vi "SLSC Update Channels State to Tree Control.vi"(0 "Property tree":refnum<vi>, 1 "Update Only?":bool, 5 "SLSC Output Tree":T1(array[cluster])=[{"Left Cell String"="SLSC-12001-030EE1BC-Mod8", "Child Text"=[], "Child Tag"="Device", "Item Indent"=0, "Child Only?"=FALSE, "Glyph Index"=28}, {"Left Cell String"="Commands", "Child Text"=[], "Child Tag"="Device/Commands", "Item Indent"=1, "Child Only?"=FALSE, "Glyph Index"=35}, {"Left Cell String"="NI.UpdateChannelConfiguration", "Child Text"=["", "", "", "", "", "", "Command..NI.UpdateChannelConfiguration", "Command to complete updating physical channel properties", "This command enables simultaneous updating of the functional state of the module's physical channel configuration. Simultaneous updating of the physical channels' properties prevents the register write commit order from creating unexpected channel configuration states. Run this command to make changes to physical channels' properties take effect."], "Child Tag"="Device/Commands/NI.UpdateChannelConfiguration", "Item Indent"=2, "Child Only?"=FALSE, "Glyph Index"=4}, {"Left Cell String"="NI.UpdateTestMode", "Child Text"=["", "", "", "", "", "", "Command..NI.UpdateTestMode", "Command to complete updating Test Mode properties", "This command enable simultaneous updating of the functional state of the module's Test Mode configuration. Run this command to make changes to Test Mode properties take effect."], "Child Tag"="Device/Commands/NI.UpdateTestMode", "Item Indent"=2, "Child Only?"=FALSE, "Glyph Index"=4}, {"Left Cell String"="NI.Acknowledge24VPowerFailed", "Child Text"=["", "", "", "", "", "", "Command..NI.Acknowledge24VPowerFailed", "Command to acknowledge a latched 24V power failure status", "This command tries to clear the module's latched true state for the NI.Status24V_PowerFailed property. This command will have no effect on the latched state if the NI.Status24V_PowerGood property is still false."], "Child Tag"="Device/Commands/NI.Acknowledge24VPowerFailed", "Item Indent"=2, "Child Only?"=FALSE, "Glyph Index"=4}, {"Left Cell String"="Properties", "Child Text"=[], "Child Tag"="Device/Properties", "Item Indent"=1, "Child Only?"=FALSE, "Glyph Index"=36}, {"Left Cell String"="NI.ModuleControllerVersion", "Child Text"=["17022812", "Read Only", "U32", "", "", "", "[3.860173E+8].R.U32..NI.ModuleControllerVersion", "Module Controller Version", "The version is the timestamp, in hexadecimal format, of the time the Module Controller was compiled."], "Child Tag"="Device/Properties/NI.ModuleControllerVersion", "Item Indent"=2, "Child Only?"=FALSE, "Glyph Index"=8}, {"Left Cell String"="NI.RearBufferState", "Child Text"=["0", "Read Only", "U32", "", "", "", "[0].R.U32..NI.RearBufferState", "Logic state of all rear I/O connector input buffers", "Reading this property retrieves the current logic state of the rear I/O connector input buffers. This retrieval is controlled through the software system so the actual sampling time of the inputs is not deterministic. The value at each bit position is a function of the logic state at the XJ2 pin and the corresponding line's direction and enable configuration. An enabled line configured as an input will drive the rear I/O connector input buffer to the same state as detected at the front I/O connector input buffer."], "Child Tag"="Device/Properties/NI.RearBufferState", "Item Indent"=2, "Child Only?"=FALSE, "Glyph Index"=8}, {"Left Cell String"="NI.FrontBufferState", "Child Text"=["0", "Read Only", "U32", "", "", "", "[0].R.U32..NI.FrontBufferState", "Logic state of all front I/O connector input buffers", "Reading this property retrieves the current logic state of the front I/O connector input buffers. This retrieval is controlled through the software system so the actual sampling time of the inputs is not deterministic. The value at each bit position is a function of the voltage at the module DSUB pin and the bank range and threshold configuration. An enabled line configured as an output may drive the front I/O connector input buffer to a specific voltage, depending on the bank supply voltage configuration, the line's output topology, and the line's logic state from the rear I/O connector input buffer."], "Child Tag"="Device/Properties/NI.FrontBufferState", "Item Indent"=2, "Child Only?"=FALSE, "Glyph Index"=8}, {"Left Cell String"="NI.Status24VPowerFailed", "Child Text"=["False", "Read Only", "Bool", "", "", "", "[0].R.Bool..NI.Status24VPowerFailed", "State of the latched failure status of the module's 24V rail from the SLSC Interface", "When the NI.Status24V_PowerGood becomes false, this property latches as true until it is reset by the NI.Status24V_FaultAcknowledge command is sent after NI.Status24V_PowerGood returns to true. If this property is true, then the supply voltage selection for both banks of the module has been forced off for a nonzero duration."], "Child Tag"="Device/Properties/NI.Status24VPowerFailed", "Item Indent"=2, "Child Only?"=FALSE, "Glyph Index"=8}, {"Left Cell String"="NI.Status24VPowerGood", "Child Text"=["True", "Read Only", "Bool", "", "", "", "[1].R.Bool..NI.Status24VPowerGood", "State of the 24V rail on the module from the SLSC Interface", "When the 24V rail from the SLSC Interface drops below the safe operating range for the module, this property is set to false. Simultaneously, to protect the module's output circuitry and to prevent the module front I/O connector outputs from glitching high, the supply voltage selection for both banks is forced off until the 24V rail recovers and is stable."], "Child Tag"="Device/Properties/NI.Status24VPowerGood", "Item Indent"=2, "Child Only?"=FALSE, "Glyph Index"=8}, {"Left Cell String"="NI.Status3_3VPowerGood", "Child Text"=["True", "Read Only", "Bool", "", "", "", "[1].R.Bool..NI.Status3_3VPowerGood", "State of the 3.3V rail from the SLSC Interface on the module", "This property will always be true on a correctly functioning module because the module CPLD requires the 3.3V rail from the SLSC Interface to operate."], "Child Tag"="Device/Properties/NI.Status3_3VPowerGood", "Item Indent"=2, "Child Only?"=FALSE, "Glyph Index"=8}, {"Left Cell String"="NI.TestModeEnable", "Child Text"=["False", "Read/Write", "Bool", "", "", "", "[0].RW.Bool..NI.TestModeEnable", "Enable for Test Mode", "Enable state for the module's Test Mode. When Test Mode is enabled, the module will output the values from the NI.TestModeValue property on the corresponding lines. Each line's respective direction and enable configuration will still apply when Test Mode is active. The data source of the lines is the only change when Test Mode is active. Changes to this property take effect after running the NI.TestModeUpdate command."], "Child Tag"="Device/Properties/NI.TestModeEnable", "Item Indent"=2, "Child Only?"=FALSE, "Glyph Index"=9}, {"Left Cell String"="NI.TestModeValue", "Child Text"=["0", "Read/Write", "U32", "", "", "", "[0].RW.U32..NI.TestModeValue", "Output logic states for use during Test Mode", "Output logic states for the module for use during Test Mode. The logic state corresponding to each line may be set independently of the other states. Changes to this property take effect after running the NI.TestModeUpdate command."], "Child Tag"="Device/Properties/NI.TestModeValue", "Item Indent"=2, "Child Only?"=FALSE, "Glyph Index"=9}, {"Left Cell String"="SLSC-12001-030EE1BC-Mod8/bank0", "Child Text"=[], "Child Tag"="Physical Channel/bank0", "Item Indent"=1, "Child Only?"=FALSE, "Glyph Index"=31}, {"Left Cell String"="Commands", "Child Text"=[], "Child Tag"="Physical Channel/bank0/Commands", "Item Indent"=2, "Child Only?"=FALSE, "Glyph Index"=35}, {"Left Cell String"="Properties", "Child Text"=[], "Child Tag"="Physical Channel/bank0/Properties", "Item Indent"=2, "Child Only?"=FALSE, "Glyph Index"=36}, {"Left Cell String"="NI.VsupSelect", "Child Text"=["[0]Vsup_Off", "Read/Write", "I32", "Enum", "NI.VsupSource", "[0]Vsup_Off;[1]Vsup_0;[2]Vsup_1;", "[0].RW.I32.bank0.NI.VsupSelect", "Voltage source selection", "Voltage source selection for this bank. Changes to this property take effect after running the NI.ChannelConfigurationUpdate command."], "Child Tag"="Physical Channel/bank0/Properties/NI.VsupSelect", "Item Indent"=3, "Child Only?"=FALSE, "Glyph Index"=9}, {"Left Cell String"="NI.RangeEnable5V", "Child Text"=["False", "Read/Write", "Bool", "", "", "", "[0].RW.Bool.bank0.NI.RangeEnable5V", "Voltage range selection", "Enable state for this bank's voltage range. When enabled, this bank uses the NI.InputThreshold5V for the input threshold. When disabled, this bank uses the NI.InputThreshold33V for the input threshold. Changes to this property take effect after running the NI.ChannelConfigurationUpdate command."], "Child Tag"="Physical Channel/bank0/Properties/NI.RangeEnable5V", "Item Indent"=3, "Child Only?"=FALSE, "Glyph Index"=9}, {"Left Cell String"="NI.InputThreshold5V", "Child Text"=["0.7", "Read/Write", "DBL", "", "", "", "[0.7].RW.DBL.bank0.NI.InputThreshold5V", "Input threshold voltage for the 5 V range", "Input threshold voltage for this bank when its NI.RangeEnable5V is true. Changes to this property take effect after running the NI.ChannelConfigurationUpdate command."], "Child Tag"="Physical Channel/bank0/Properties/NI.InputThreshold5V", "Item Indent"=3, "Child Only?"=FALSE, "Glyph Index"=9}, {"Left Cell String"="NI.InputThreshold33V", "Child Text"=["3.706", "Read/Write", "DBL", "", "", "", "[3.706].RW.DBL.bank0.NI.InputThreshold33V", "Input threshold voltage for the 33 V range", "Input threshold voltage for this bank when its NI.RangeEnable5V is false. Changes to this property take effect after running the NI.ChannelConfigurationUpdate command."], "Child Tag"="Physical Channel/bank0/Properties/NI.InputThreshold33V", "Item Indent"=3, "Child Only?"=FALSE, "Glyph Index"=9}, {"Left Cell String"="SLSC-12001-030EE1BC-Mod8/bank1", "Child Text"=[], "Child Tag"="Physical Channel/bank1", "Item Indent"=1, "Child Only?"=FALSE, "Glyph Index"=31}, {"Left Cell String"="Commands", "Child Text"=[], "Child Tag"="Physical Channel/bank1/Commands", "Item Indent"=2, "Child Only?"=FALSE, "Glyph Index"=35}, {"Left Cell String"="Properties", "Child Text"=[], "Child Tag"="Physical Channel/bank1/Properties", "Item Indent"=2, "Child Only?"=FALSE, "Glyph Index"=36}, {"Left Cell String"="NI.VsupSelect", "Child Text"=["[0]Vsup_Off", "Read/Write", "I32", "Enum", "NI.VsupSource", "[0]Vsup_Off;[1]Vsup_0;[2]Vsup_1;", "[0].RW.I32.bank1.NI.VsupSelect", "Voltage source selection", "Voltage source selection for this bank. Changes to this property take effect after running the NI.ChannelConfigurationUpdate command."], "Child Tag"="Physical Channel/bank1/Properties/NI.VsupSelect", "Item Indent"=3, "Child Only?"=FALSE, "Glyph Index"=9}, {"Left Cell String"="NI.RangeEnable5V", "Child Text"=["False", "Read/Write", "Bool", "", "", "", "[0].RW.Bool.bank1.NI.RangeEnable5V", "Voltage range selection", "Enable state for this bank's voltage range. When enabled, this bank uses the NI.InputThreshold5V for the input threshold. When disabled, this bank uses the NI.InputThreshold33V for the input threshold. Changes to this property take effect after running the NI.ChannelConfigurationUpdate command."], "Child Tag"="Physical Channel/bank1/Properties/NI.RangeEnable5V", "Item Indent"=3, "Child Only?"=FALSE, "Glyph Index"=9}, {"Left Cell String"="NI.InputThreshold5V", "Child Text"=["0.7", "Read/Write", "DBL", "", "", "", "[0.7].RW.DBL.bank1.NI.InputThreshold5V", "Input threshold voltage for the 5 V range", "Input threshold voltage for this bank when its NI.RangeEnable5V is true. Changes to this property take effect after running the NI.ChannelConfigurationUpdate command."], "Child Tag"="Physical Channel/bank1/Properties/NI.InputThreshold5V", "Item Indent"=3, "Child Only?"=FALSE, "Glyph Index"=9}, {"Left Cell String"="NI.InputThreshold33V", "Child Text"=["3.706", "Read/Write", "DBL", "", "", "", "[3.706].RW.DBL.bank1.NI.InputThreshold33V", "Input threshold voltage for the 33 V range", "Input threshold voltage for this bank when its NI.RangeEnable5V is false. Changes to this property take effect after running the NI.ChannelConfigurationUpdate command."], "Child Tag"="Physical Channel/bank1/Properties/NI.InputThreshold33V", "Item Indent"=3, "Child Only?"=FALSE, "Glyph Index"=9}, {"Left Cell String"="SLSC-12001-030EE1BC-Mod8/port0/line0", "Child Text"=[], "Child Tag"="Physical Channel/port0/line0", "Item Indent"=1, "Child Only?"=FALSE, "Glyph Index"=31}, {"Left Cell String"="Commands", "Child Text"=[], "Child Tag"="Physical Channel/port0/line0/Commands", "Item Indent"=2, "Child Only?"=FALSE, "Glyph Index"=35}, {"Left Cell String"="Properties", "Child Text"=[], "Child Tag"="Physical Channel/port0/line0/Properties", "Item Indent"=2, "Child Only?"=FALSE, "Glyph Index"=36}, {"Left Cell String"="NI.Line.Index", "Child Text"=["0", "Read Only", "U32", "", "", "", "[0].R.U32.port0/line0.NI.Line.Index", "Overall index of this DIO line in the module", "This is the index of this DIO line for the aggregate module properties: NI.FrontInputBufferState, NI.RearInputBufferState, and NI.TestModeValue."], "Child Tag"="Physical Channel/port0/line0/Properties/NI.Line.Index", "Item Indent"=3, "Child Only?"=FALSE, "Glyph Index"=8}, {"Left Cell String"="NI.Line.Direction", "Child Text"=["[0]Input", "Read/Write", "I32", "Enum", "NI.Line.Direction", "[0]Input;[1]Output_Source;[2]Output_Sink;[3]Output_PushPull;", "[0].RW.I32.port0/line0.NI.Line.Direction", "DIO line direction", "Line signal flow direction through the module, relative to the front I/O connector. This property is only used when the NI.ChannelEnable for this line is set to true. Changes to this property take effect after running the NI.ChannelConfigurationUpdate command."], "Child Tag"="Physical Channel/port0/line0/Properties/NI.Line.Direction", "Item Indent"=3, "Child Only?"=FALSE, "Glyph Index"=9}, {"Left Cell String"="NI.Line.Enable", "Child Text"=["False", "Read/Write", "Bool", "", "", "", "[0].RW.Bool.port0/line0.NI.Line.Enable", "DIO line output enable", "DIO output enable for one line. When a line is enabled, the input and output buffers for the front I/O connector and the rear I/O connector of the line are configured based on the NI.Line.Direction property. When a line is not enabled, the buffers for both the front I/O connector and the rear I/O connector are configured as inputs. Changes to this property take effect after running the NI.ChannelConfigurationUpdate command."], "Child Tag"="Physical Channel/port0/line0/Properties/NI.Line.Enable", "Item Indent"=3, "Child Only?"=FALSE, "Glyph Index"=9}, {"Left Cell String"="SLSC-12001-030EE1BC-Mod8/port0/line1", "Child Text"=[], "Child Tag"="Physical Channel/port0/line1", "Item Indent"=1, "Child Only?"=FALSE, "Glyph Index"=31}, {"Left Cell String"="Commands", "Child Text"=[], "Child Tag"="Physical Channel/port0/line1/Commands", "Item Indent"=2, "Child Only?"=FALSE, "Glyph Index"=35}, {"Left Cell String"="Properties", "Child Text"=[], "Child Tag"="Physical Channel/port0/line1/Properties", "Item Indent"=2, "Child Only?"=FALSE, "Glyph Index"=36}, {"Left Cell String"="NI.Line.Index", "Child Text"=["1", "Read Only", "U32", "", "", "", "[1].R.U32.port0/line1.NI.Line.Index", "Overall index of this DIO line in the module", "This is the index of this DIO line for the aggregate module properties: NI.FrontInputBufferState, NI.RearInputBufferState, and NI.TestModeValue."], "Child Tag"="Physical Channel/port0/line1/Properties/NI.Line.Index", "Item Indent"=3, "Child Only?"=FALSE, "Glyph Index"=8}, {"Left Cell String"="NI.Line.Direction", "Child Text"=["[0]Input", "Read/Write", "I32", "Enum", "NI.Line.Direction", "[0]Input;[1]Output_Source;[2]Output_Sink;[3]Output_PushPull;", "[0].RW.I32.port0/line1.NI.Line.Direction", "DIO line direction", "Line signal flow direction through the module, relative to the front I/O connector. This property is only used when the NI.ChannelEnable for this line is set to true. Changes to this property take effect after running the NI.ChannelConfigurationUpdate command."], "Child Tag"="Physical Channel/port0/line1/Properties/NI.Line.Direction", "Item Indent"=3, "Child Only?"=FALSE, "Glyph Index"=9}, {"Left Cell String"="NI.Line.Enable", "Child Text"=["False", "Read/Write", "Bool", "", "", "", "[0].RW.Bool.port0/line1.NI.Line.Enable", "DIO line output enable", "DIO output enable for one line. When a line is enabled, the input and output buffers for the front I/O connector and the rear I/O connector of the line are configured based on the NI.Line.Direction property. When a line is not enabled, the buffers for both the front I/O connector and the rear I/O connector are configured as inputs. Changes to this property take effect after running the NI.ChannelConfigurationUpdate command."], "Child Tag"="Physical Channel/port0/line1/Properties/NI.Line.Enable", "Item Indent"=3, "Child Only?"=FALSE, "Glyph Index"=9}, {"Left Cell String"="SLSC-12001-030EE1BC-Mod8/port0/line2", "Child Text"=[], "Child Tag"="Physical Channel/port0/line2", "Item Indent"=1, "Child Only?"=FALSE, "Glyph Index"=31}, {"Left Cell String"="Commands", "Child Text"=[], "Child Tag"="Physical Channel/port0/line2/Commands", "Item Indent"=2, "Child Only?"=FALSE, "Glyph Index"=35}, {"Left Cell String"="Properties", "Child Text"=[], "Child Tag"="Physical Channel/port0/line2/Properties", "Item Indent"=2, "Child Only?"=FALSE, "Glyph Index"=36}, {"Left Cell String"="NI.Line.Index", "Child Text"=["2", "Read Only", "U32", "", "", "", "[2].R.U32.port0/line2.NI.Line.Index", "Overall index of this DIO line in the module", "This is the index of this DIO line for the aggregate module properties: NI.FrontInputBufferState, NI.RearInputBufferState, and NI.TestModeValue."], "Child Tag"="Physical Channel/port0/line2/Properties/NI.Line.Index", "Item Indent"=3, "Child Only?"=FALSE, "Glyph Index"=8}, {"Left Cell String"="NI.Line.Direction", "Child Text"=["[0]Input", "Read/Write", "I32", "Enum", "NI.Line.Direction", "[0]Input;[1]Output_Source;[2]Output_Sink;[3]Output_PushPull;", "[0].RW.I32.port0/line2.NI.Line.Direction", "DIO line direction", "Line signal flow direction through the module, relative to the front I/O connector. This property is only used when the NI.ChannelEnable for this line is set to true. Changes to this property take effect after running the NI.ChannelConfigurationUpdate command."], "Child Tag"="Physical Channel/port0/line2/Properties/NI.Line.Direction", "Item Indent"=3, "Child Only?"=FALSE, "Glyph Index"=9}, {"Left Cell String"="NI.Line.Enable", "Child Text"=["False", "Read/Write", "Bool", "", "", "", "[0].RW.Bool.port0/line2.NI.Line.Enable", "DIO line output enable", "DIO output enable for one line. When a line is enabled, the input and output buffers for the front I/O connector and the rear I/O connector of the line are configured based on the NI.Line.Direction property. When a line is not enabled, the buffers for both the front I/O connector and the rear I/O connector are configured as inputs. Changes to this property take effect after running the NI.ChannelConfigurationUpdate command."], "Child Tag"="Physical Channel/port0/line2/Properties/NI.Line.Enable", "Item Indent"=3, "Child Only?"=FALSE, "Glyph Index"=9}, {"Left Cell String"="SLSC-12001-030EE1BC-Mod8/port0/line3", "Child Text"=[], "Child Tag"="Physical Channel/port0/line3", "Item Indent"=1, "Child Only?"=FALSE, "Glyph Index"=31}, {"Left Cell String"="Commands", "Child Text"=[], "Child Tag"="Physical Channel/port0/line3/Commands", "Item Indent"=2, "Child Only?"=FALSE, "Glyph Index"=35}, {"Left Cell String"="Properties", "Child Text"=[], "Child Tag"="Physical Channel/port0/line3/Properties", "Item Indent"=2, "Child Only?"=FALSE, "Glyph Index"=36}, {"Left Cell String"="NI.Line.Index", "Child Text"=["3", "Read Only", "U32", "", "", "", "[3].R.U32.port0/line3.NI.Line.Index", "Overall index of this DIO line in the module", "This is the index of this DIO line for the aggregate module properties: NI.FrontInputBufferState, NI.RearInputBufferState, and NI.TestModeValue."], "Child Tag"="Physical Channel/port0/line3/Properties/NI.Line.Index", "Item Indent"=3, "Child Only?"=FALSE, "Glyph Index"=8}, {"Left Cell String"="NI.Line.Direction", "Child Text"=["[0]Input", "Read/Write", "I32", "Enum", "NI.Line.Direction", "[0]Input;[1]Output_Source;[2]Output_Sink;[3]Output_PushPull;", "[0].RW.I32.port0/line3.NI.Line.Direction", "DIO line direction", "Line signal flow direction through the module, relative to the front I/O connector. This property is only used when the NI.ChannelEnable for this line is set to true. Changes to this property take effect after running the NI.ChannelConfigurationUpdate command."], "Child Tag"="Physical Channel/port0/line3/Properties/NI.Line.Direction", "Item Indent"=3, "Child Only?"=FALSE, "Glyph Index"=9}, {"Left Cell String"="NI.Line.Enable", "Child Text"=["False", "Read/Write", "Bool", "", "", "", "[0].RW.Bool.port0/line3.NI.Line.Enable", "DIO line output enable", "DIO output enable for one line. When a line is enabled, the input and output buffers for the front I/O connector and the rear I/O connector of the line are configured based on the NI.Line.Direction property. When a line is not enabled, the buffers for both the front I/O connector and the rear I/O connector are configured as inputs. Changes to this property take effect after running the NI.ChannelConfigurationUpdate command."], "Child Tag"="Physical Channel/port0/line3/Properties/NI.Line.Enable", "Item Indent"=3, "Child Only?"=FALSE, "Glyph Index"=9}, {"Left Cell String"="SLSC-12001-030EE1BC-Mod8/port0/line4", "Child Text"=[], "Child Tag"="Physical Channel/port0/line4", "Item Indent"=1, "Child Only?"=FALSE, "Glyph Index"=31}, {"Left Cell String"="Commands", "Child Text"=[], "Child Tag"="Physical Channel/port0/line4/Commands", "Item Indent"=2, "Child Only?"=FALSE, "Glyph Index"=35}, {"Left Cell String"="Properties", "Child Text"=[], "Child Tag"="Physical Channel/port0/line4/Properties", "Item Indent"=2, "Child Only?"=FALSE, "Glyph Index"=36}, {"Left Cell String"="NI.Line.Index", "Child Text"=["4", "Read Only", "U32", "", "", "", "[4].R.U32.port0/line4.NI.Line.Index", "Overall index of this DIO line in the module", "This is the index of this DIO line for the aggregate module properties: NI.FrontInputBufferState, NI.RearInputBufferState, and NI.TestModeValue."], "Child Tag"="Physical Channel/port0/line4/Properties/NI.Line.Index", "Item Indent"=3, "Child Only?"=FALSE, "Glyph Index"=8}, {"Left Cell String"="NI.Line.Direction", "Child Text"=["[0]Input", "Read/Write", "I32", "Enum", "NI.Line.Direction", "[0]Input;[1]Output_Source;[2]Output_Sink;[3]Output_PushPull;", "[0].RW.I32.port0/line4.NI.Line.Direction", "DIO line direction", "Line signal flow direction through the module, relative to the front I/O connector. This property is only used when the NI.ChannelEnable for this line is set to true. Changes to this property take effect after running the NI.ChannelConfigurationUpdate command."], "Child Tag"="Physical Channel/port0/line4/Properties/NI.Line.Direction", "Item Indent"=3, "Child Only?"=FALSE, "Glyph Index"=9}, {"Left Cell String"="NI.Line.Enable", "Child Text"=["False", "Read/Write", "Bool", "", "", "", "[0].RW.Bool.port0/line4.NI.Line.Enable", "DIO line output enable", "DIO output enable for one line. When a line is enabled, the input and output buffers for the front I/O connector and the rear I/O connector of the line are configured based on the NI.Line.Direction property. When a line is not enabled, the buffers for both the front I/O connector and the rear I/O connector are configured as inputs. Changes to this property take effect after running the NI.ChannelConfigurationUpdate command."], "Child Tag"="Physical Channel/port0/line4/Properties/NI.Line.Enable", "Item Indent"=3, "Child Only?"=FALSE, "Glyph Index"=9}, {"Left Cell String"="SLSC-12001-030EE1BC-Mod8/port0/line5", "Child Text"=[], "Child Tag"="Physical Channel/port0/line5", "Item Indent"=1, "Child Only?"=FALSE, "Glyph Index"=31}, {"Left Cell String"="Commands", "Child Text"=[], "Child Tag"="Physical Channel/port0/line5/Commands", "Item Indent"=2, "Child Only?"=FALSE, "Glyph Index"=35}, {"Left Cell String"="Properties", "Child Text"=[], "Child Tag"="Physical Channel/port0/line5/Properties", "Item Indent"=2, "Child Only?"=FALSE, "Glyph Index"=36}, {"Left Cell String"="NI.Line.Index", "Child Text"=["5", "Read Only", "U32", "", "", "", "[5].R.U32.port0/line5.NI.Line.Index", "Overall index of this DIO line in the module", "This is the index of this DIO line for the aggregate module properties: NI.FrontInputBufferState, NI.RearInputBufferState, and NI.TestModeValue."], "Child Tag"="Physical Channel/port0/line5/Properties/NI.Line.Index", "Item Indent"=3, "Child Only?"=FALSE, "Glyph Index"=8}, {"Left Cell String"="NI.Line.Direction", "Child Text"=["[0]Input", "Read/Write", "I32", "Enum", "NI.Line.Direction", "[0]Input;[1]Output_Source;[2]Output_Sink;[3]Output_PushPull;", "[0].RW.I32.port0/line5.NI.Line.Direction", "DIO line direction", "Line signal flow direction through the module, relative to the front I/O connector. This property is only used when the NI.ChannelEnable for this line is set to true. Changes to this property take effect after running the NI.ChannelConfigurationUpdate command."], "Child Tag"="Physical Channel/port0/line5/Properties/NI.Line.Direction", "Item Indent"=3, "Child Only?"=FALSE, "Glyph Index"=9}, {"Left Cell String"="NI.Line.Enable", "Child Text"=["False", "Read/Write", "Bool", "", "", "", "[0].RW.Bool.port0/line5.NI.Line.Enable", "DIO line output enable", "DIO output enable for one line. When a line is enabled, the input and output buffers for the front I/O connector and the rear I/O connector of the line are configured based on the NI.Line.Direction property. When a line is not enabled, the buffers for both the front I/O connector and the rear I/O connector are configured as inputs. Changes to this property take effect after running the NI.ChannelConfigurationUpdate command."], "Child Tag"="Physical Channel/port0/line5/Properties/NI.Line.Enable", "Item Indent"=3, "Child Only?"=FALSE, "Glyph Index"=9}, {"Left Cell String"="SLSC-12001-030EE1BC-Mod8/port0/line6", "Child Text"=[], "Child Tag"="Physical Channel/port0/line6", "Item Indent"=1, "Child Only?"=FALSE, "Glyph Index"=31}, {"Left Cell String"="Commands", "Child Text"=[], "Child Tag"="Physical Channel/port0/line6/Commands", "Item Indent"=2, "Child Only?"=FALSE, "Glyph Index"=35}, {"Left Cell String"="Properties", "Child Text"=[], "Child Tag"="Physical Channel/port0/line6/Properties", "Item Indent"=2, "Child Only?"=FALSE, "Glyph Index"=36}, {"Left Cell String"="NI.Line.Index", "Child Text"=["6", "Read Only", "U32", "", "", "", "[6].R.U32.port0/line6.NI.Line.Index", "Overall index of this DIO line in the module", "This is the index of this DIO line for the aggregate module properties: NI.FrontInputBufferState, NI.RearInputBufferState, and NI.TestModeValue."], "Child Tag"="Physical Channel/port0/line6/Properties/NI.Line.Index", "Item Indent"=3, "Child Only?"=FALSE, "Glyph Index"=8}, {"Left Cell String"="NI.Line.Direction", "Child Text"=["[0]Input", "Read/Write", "I32", "Enum", "NI.Line.Direction", "[0]Input;[1]Output_Source;[2]Output_Sink;[3]Output_PushPull;", "[0].RW.I32.port0/line6.NI.Line.Direction", "DIO line direction", "Line signal flow direction through the module, relative to the front I/O connector. This property is only used when the NI.ChannelEnable for this line is set to true. Changes to this property take effect after running the NI.ChannelConfigurationUpdate command."], "Child Tag"="Physical Channel/port0/line6/Properties/NI.Line.Direction", "Item Indent"=3, "Child Only?"=FALSE, "Glyph Index"=9}, {"Left Cell String"="NI.Line.Enable", "Child Text"=["False", "Read/Write", "Bool", "", "", "", "[0].RW.Bool.port0/line6.NI.Line.Enable", "DIO line output enable", "DIO output enable for one line. When a line is enabled, the input and output buffers for the front I/O connector and the rear I/O connector of the line are configured based on the NI.Line.Direction property. When a line is not enabled, the buffers for both the front I/O connector and the rear I/O connector are configured as inputs. Changes to this property take effect after running the NI.ChannelConfigurationUpdate command."], "Child Tag"="Physical Channel/port0/line6/Properties/NI.Line.Enable", "Item Indent"=3, "Child Only?"=FALSE, "Glyph Index"=9}, {"Left Cell String"="SLSC-12001-030EE1BC-Mod8/port0/line7", "Child Text"=[], "Child Tag"="Physical Channel/port0/line7", "Item Indent"=1, "Child Only?"=FALSE, "Glyph Index"=31}, {"Left Cell String"="Commands", "Child Text"=[], "Child Tag"="Physical Channel/port0/line7/Commands", "Item Indent"=2, "Child Only?"=FALSE, "Glyph Index"=35}, {"Left Cell String"="Properties", "Child Text"=[], "Child Tag"="Physical Channel/port0/line7/Properties", "Item Indent"=2, "Child Only?"=FALSE, "Glyph Index"=36}, {"Left Cell String"="NI.Line.Index", "Child Text"=["7", "Read Only", "U32", "", "", "", "[7].R.U32.port0/line7.NI.Line.Index", "Overall index of this DIO line in the module", "This is the index of this DIO line for the aggregate module properties: NI.FrontInputBufferState, NI.RearInputBufferState, and NI.TestModeValue."], "Child Tag"="Physical Channel/port0/line7/Properties/NI.Line.Index", "Item Indent"=3, "Child Only?"=FALSE, "Glyph Index"=8}, {"Left Cell String"="NI.Line.Direction", "Child Text"=["[0]Input", "Read/Write", "I32", "Enum", "NI.Line.Direction", "[0]Input;[1]Output_Source;[2]Output_Sink;[3]Output_PushPull;", "[0].RW.I32.port0/line7.NI.Line.Direction", "DIO line direction", "Line signal flow direction through the module, relative to the front I/O connector. This property is only used when the NI.ChannelEnable for this line is set to true. Changes to this property take effect after running the NI.ChannelConfigurationUpdate command."], "Child Tag"="Physical Channel/port0/line7/Properties/NI.Line.Direction", "Item Indent"=3, "Child Only?"=FALSE, "Glyph Index"=9}, {"Left Cell String"="NI.Line.Enable", "Child Text"=["False", "Read/Write", "Bool", "", "", "", "[0].RW.Bool.port0/line7.NI.Line.Enable", "DIO line output enable", "DIO output enable for one line. When a line is enabled, the input and output buffers for the front I/O connector and the rear I/O connector of the line are configured based on the NI.Line.Direction property. When a line is not enabled, the buffers for both the front I/O connector and the rear I/O connector are configured as inputs. Changes to this property take effect after running the NI.ChannelConfigurationUpdate command."], "Child Tag"="Physical Channel/port0/line7/Properties/NI.Line.Enable", "Item Indent"=3, "Child Only?"=FALSE, "Glyph Index"=9}, {"Left Cell String"="SLSC-12001-030EE1BC-Mod8/port1/line0", "Child Text"=[], "Child Tag"="Physical Channel/port1/line0", "Item Indent"=1, "Child Only?"=FALSE, "Glyph Index"=31}, {"Left Cell String"="Commands", "Child Text"=[], "Child Tag"="Physical Channel/port1/line0/Commands", "Item Indent"=2, "Child Only?"=FALSE, "Glyph Index"=35}, {"Left Cell String"="Properties", "Child Text"=[], "Child Tag"="Physical Channel/port1/line0/Properties", "Item Indent"=2, "Child Only?"=FALSE, "Glyph Index"=36}, {"Left Cell String"="NI.Line.Index", "Child Text"=["8", "Read Only", "U32", "", "", "", "[8].R.U32.port1/line0.NI.Line.Index", "Overall index of this DIO line in the module", "This is the index of this DIO line for the aggregate module properties: NI.FrontInputBufferState, NI.RearInputBufferState, and NI.TestModeValue."], "Child Tag"="Physical Channel/port1/line0/Properties/NI.Line.Index", "Item Indent"=3, "Child Only?"=FALSE, "Glyph Index"=8}, {"Left Cell String"="NI.Line.Direction", "Child Text"=["[0]Input", "Read/Write", "I32", "Enum", "NI.Line.Direction", "[0]Input;[1]Output_Source;[2]Output_Sink;[3]Output_PushPull;", "[0].RW.I32.port1/line0.NI.Line.Direction", "DIO line direction", "Line signal flow direction through the module, relative to the front I/O connector. This property is only used when the NI.ChannelEnable for this line is set to true. Changes to this property take effect after running the NI.ChannelConfigurationUpdate command."], "Child Tag"="Physical Channel/port1/line0/Properties/NI.Line.Direction", "Item Indent"=3, "Child Only?"=FALSE, "Glyph Index"=9}, {"Left Cell String"="NI.Line.Enable", "Child Text"=["False", "Read/Write", "Bool", "", "", "", "[0].RW.Bool.port1/line0.NI.Line.Enable", "DIO line output enable", "DIO output enable for one line. When a line is enabled, the input and output buffers for the front I/O connector and the rear I/O connector of the line are configured based on the NI.Line.Direction property. When a line is not enabled, the buffers for both the front I/O connector and the rear I/O connector are configured as inputs. Changes to this property take effect after running the NI.ChannelConfigurationUpdate command."], "Child Tag"="Physical Channel/port1/line0/Properties/NI.Line.Enable", "Item Indent"=3, "Child Only?"=FALSE, "Glyph Index"=9}, {"Left Cell String"="SLSC-12001-030EE1BC-Mod8/port1/line1", "Child Text"=[], "Child Tag"="Physical Channel/port1/line1", "Item Indent"=1, "Child Only?"=FALSE, "Glyph Index"=31}, {"Left Cell String"="Commands", "Child Text"=[], "Child Tag"="Physical Channel/port1/line1/Commands", "Item Indent"=2, "Child Only?"=FALSE, "Glyph Index"=35}, {"Left Cell String"="Properties", "Child Text"=[], "Child Tag"="Physical Channel/port1/line1/Properties", "Item Indent"=2, "Child Only?"=FALSE, "Glyph Index"=36}, {"Left Cell String"="NI.Line.Index", "Child Text"=["9", "Read Only", "U32", "", "", "", "[9].R.U32.port1/line1.NI.Line.Index", "Overall index of this DIO line in the module", "This is the index of this DIO line for the aggregate module properties: NI.FrontInputBufferState, NI.RearInputBufferState, and NI.TestModeValue."], "Child Tag"="Physical Channel/port1/line1/Properties/NI.Line.Index", "Item Indent"=3, "Child Only?"=FALSE, "Glyph Index"=8}, {"Left Cell String"="NI.Line.Direction", "Child Text"=["[0]Input", "Read/Write", "I32", "Enum", "NI.Line.Direction", "[0]Input;[1]Output_Source;[2]Output_Sink;[3]Output_PushPull;", "[0].RW.I32.port1/line1.NI.Line.Direction", "DIO line direction", "Line signal flow direction through the module, relative to the front I/O connector. This property is only used when the NI.ChannelEnable for this line is set to true. Changes to this property take effect after running the NI.ChannelConfigurationUpdate command."], "Child Tag"="Physical Channel/port1/line1/Properties/NI.Line.Direction", "Item Indent"=3, "Child Only?"=FALSE, "Glyph Index"=9}, {"Left Cell String"="NI.Line.Enable", "Child Text"=["False", "Read/Write", "Bool", "", "", "", "[0].RW.Bool.port1/line1.NI.Line.Enable", "DIO line output enable", "DIO output enable for one line. When a line is enabled, the input and output buffers for the front I/O connector and the rear I/O connector of the line are configured based on the NI.Line.Direction property. When a line is not enabled, the buffers for both the front I/O connector and the rear I/O connector are configured as inputs. Changes to this property take effect after running the NI.ChannelConfigurationUpdate command."], "Child Tag"="Physical Channel/port1/line1/Properties/NI.Line.Enable", "Item Indent"=3, "Child Only?"=FALSE, "Glyph Index"=9}, {"Left Cell String"="SLSC-12001-030EE1BC-Mod8/port1/line2", "Child Text"=[], "Child Tag"="Physical Channel/port1/line2", "Item Indent"=1, "Child Only?"=FALSE, "Glyph Index"=31}, {"Left Cell String"="Commands", "Child Text"=[], "Child Tag"="Physical Channel/port1/line2/Commands", "Item Indent"=2, "Child Only?"=FALSE, "Glyph Index"=35}, {"Left Cell String"="Properties", "Child Text"=[], "Child Tag"="Physical Channel/port1/line2/Properties", "Item Indent"=2, "Child Only?"=FALSE, "Glyph Index"=36}, {"Left Cell String"="NI.Line.Index", "Child Text"=["A", "Read Only", "U32", "", "", "", "[10].R.U32.port1/line2.NI.Line.Index", "Overall index of this DIO line in the module", "This is the index of this DIO line for the aggregate module properties: NI.FrontInputBufferState, NI.RearInputBufferState, and NI.TestModeValue."], "Child Tag"="Physical Channel/port1/line2/Properties/NI.Line.Index", "Item Indent"=3, "Child Only?"=FALSE, "Glyph Index"=8}, {"Left Cell String"="NI.Line.Direction", "Child Text"=["[0]Input", "Read/Write", "I32", "Enum", "NI.Line.Direction", "[0]Input;[1]Output_Source;[2]Output_Sink;[3]Output_PushPull;", "[0].RW.I32.port1/line2.NI.Line.Direction", "DIO line direction", "Line signal flow direction through the module, relative to the front I/O connector. This property is only used when the NI.ChannelEnable for this line is set to true. Changes to this property take effect after running the NI.ChannelConfigurationUpdate command."], "Child Tag"="Physical Channel/port1/line2/Properties/NI.Line.Direction", "Item Indent"=3, "Child Only?"=FALSE, "Glyph Index"=9}, {"Left Cell String"="NI.Line.Enable", "Child Text"=["False", "Read/Write", "Bool", "", "", "", "[0].RW.Bool.port1/line2.NI.Line.Enable", "DIO line output enable", "DIO output enable for one line. When a line is enabled, the input and output buffers for the front I/O connector and the rear I/O connector of the line are configured based on the NI.Line.Direction property. When a line is not enabled, the buffers for both the front I/O connector and the rear I/O connector are configured as inputs. Changes to this property take effect after running the NI.ChannelConfigurationUpdate command."], "Child Tag"="Physical Channel/port1/line2/Properties/NI.Line.Enable", "Item Indent"=3, "Child Only?"=FALSE, "Glyph Index"=9}, {"Left Cell String"="SLSC-12001-030EE1BC-Mod8/port1/line3", "Child Text"=[], "Child Tag"="Physical Channel/port1/line3", "Item Indent"=1, "Child Only?"=FALSE, "Glyph Index"=31}, {"Left Cell String"="Commands", "Child Text"=[], "Child Tag"="Physical Channel/port1/line3/Commands", "Item Indent"=2, "Child Only?"=FALSE, "Glyph Index"=35}, {"Left Cell String"="Properties", "Child Text"=[], "Child Tag"="Physical Channel/port1/line3/Properties", "Item Indent"=2, "Child Only?"=FALSE, "Glyph Index"=36}, {"Left Cell String"="NI.Line.Index", "Child Text"=["B", "Read Only", "U32", "", "", "", "[11].R.U32.port1/line3.NI.Line.Index", "Overall index of this DIO line in the module", "This is the index of this DIO line for the aggregate module properties: NI.FrontInputBufferState, NI.RearInputBufferState, and NI.TestModeValue."], "Child Tag"="Physical Channel/port1/line3/Properties/NI.Line.Index", "Item Indent"=3, "Child Only?"=FALSE, "Glyph Index"=8}, {"Left Cell String"="NI.Line.Direction", "Child Text"=["[0]Input", "Read/Write", "I32", "Enum", "NI.Line.Direction", "[0]Input;[1]Output_Source;[2]Output_Sink;[3]Output_PushPull;", "[0].RW.I32.port1/line3.NI.Line.Direction", "DIO line direction", "Line signal flow direction through the module, relative to the front I/O connector. This property is only used when the NI.ChannelEnable for this line is set to true. Changes to this property take effect after running the NI.ChannelConfigurationUpdate command."], "Child Tag"="Physical Channel/port1/line3/Properties/NI.Line.Direction", "Item Indent"=3, "Child Only?"=FALSE, "Glyph Index"=9}, {"Left Cell String"="NI.Line.Enable", "Child Text"=["False", "Read/Write", "Bool", "", "", "", "[0].RW.Bool.port1/line3.NI.Line.Enable", "DIO line output enable", "DIO output enable for one line. When a line is enabled, the input and output buffers for the front I/O connector and the rear I/O connector of the line are configured based on the NI.Line.Direction property. When a line is not enabled, the buffers for both the front I/O connector and the rear I/O connector are configured as inputs. Changes to this property take effect after running the NI.ChannelConfigurationUpdate command."], "Child Tag"="Physical Channel/port1/line3/Properties/NI.Line.Enable", "Item Indent"=3, "Child Only?"=FALSE, "Glyph Index"=9}, {"Left Cell String"="SLSC-12001-030EE1BC-Mod8/port1/line4", "Child Text"=[], "Child Tag"="Physical Channel/port1/line4", "Item Indent"=1, "Child Only?"=FALSE, "Glyph Index"=31}, {"Left Cell String"="Commands", "Child Text"=[], "Child Tag"="Physical Channel/port1/line4/Commands", "Item Indent"=2, "Child Only?"=FALSE, "Glyph Index"=35}, {"Left Cell String"="Properties", "Child Text"=[], "Child Tag"="Physical Channel/port1/line4/Properties", "Item Indent"=2, "Child Only?"=FALSE, "Glyph Index"=36}, {"Left Cell String"="NI.Line.Index", "Child Text"=["C", "Read Only", "U32", "", "", "", "[12].R.U32.port1/line4.NI.Line.Index", "Overall index of this DIO line in the module", "This is the index of this DIO line for the aggregate module properties: NI.FrontInputBufferState, NI.RearInputBufferState, and NI.TestModeValue."], "Child Tag"="Physical Channel/port1/line4/Properties/NI.Line.Index", "Item Indent"=3, "Child Only?"=FALSE, "Glyph Index"=8}, {"Left Cell String"="NI.Line.Direction", "Child Text"=["[0]Input", "Read/Write", "I32", "Enum", "NI.Line.Direction", "[0]Input;[1]Output_Source;[2]Output_Sink;[3]Output_PushPull;", "[0].RW.I32.port1/line4.NI.Line.Direction", "DIO line direction", "Line signal flow direction through the module, relative to the front I/O connector. This property is only used when the NI.ChannelEnable for this line is set to true. Changes to this property take effect after running the NI.ChannelConfigurationUpdate command."], "Child Tag"="Physical Channel/port1/line4/Properties/NI.Line.Direction", "Item Indent"=3, "Child Only?"=FALSE, "Glyph Index"=9}, {"Left Cell String"="NI.Line.Enable", "Child Text"=["False", "Read/Write", "Bool", "", "", "", "[0].RW.Bool.port1/line4.NI.Line.Enable", "DIO line output enable", "DIO output enable for one line. When a line is enabled, the input and output buffers for the front I/O connector and the rear I/O connector of the line are configured based on the NI.Line.Direction property. When a line is not enabled, the buffers for both the front I/O connector and the rear I/O connector are configured as inputs. Changes to this property take effect after running the NI.ChannelConfigurationUpdate command."], "Child Tag"="Physical Channel/port1/line4/Properties/NI.Line.Enable", "Item Indent"=3, "Child Only?"=FALSE, "Glyph Index"=9}, {"Left Cell String"="SLSC-12001-030EE1BC-Mod8/port1/line5", "Child Text"=[], "Child Tag"="Physical Channel/port1/line5", "Item Indent"=1, "Child Only?"=FALSE, "Glyph Index"=31}, {"Left Cell String"="Commands", "Child Text"=[], "Child Tag"="Physical Channel/port1/line5/Commands", "Item Indent"=2, "Child Only?"=FALSE, "Glyph Index"=35}, {"Left Cell String"="Properties", "Child Text"=[], "Child Tag"="Physical Channel/port1/line5/Properties", "Item Indent"=2, "Child Only?"=FALSE, "Glyph Index"=36}, {"Left Cell String"="NI.Line.Index", "Child Text"=["D", "Read Only", "U32", "", "", "", "[13].R.U32.port1/line5.NI.Line.Index", "Overall index of this DIO line in the module", "This is the index of this DIO line for the aggregate module properties: NI.FrontInputBufferState, NI.RearInputBufferState, and NI.TestModeValue."], "Child Tag"="Physical Channel/port1/line5/Properties/NI.Line.Index", "Item Indent"=3, "Child Only?"=FALSE, "Glyph Index"=8}, {"Left Cell String"="NI.Line.Direction", "Child Text"=["[0]Input", "Read/Write", "I32", "Enum", "NI.Line.Direction", "[0]Input;[1]Output_Source;[2]Output_Sink;[3]Output_PushPull;", "[0].RW.I32.port1/line5.NI.Line.Direction", "DIO line direction", "Line signal flow direction through the module, relative to the front I/O connector. This property is only used when the NI.ChannelEnable for this line is set to true. Changes to this property take effect after running the NI.ChannelConfigurationUpdate command."], "Child Tag"="Physical Channel/port1/line5/Properties/NI.Line.Direction", "Item Indent"=3, "Child Only?"=FALSE, "Glyph Index"=9}, {"Left Cell String"="NI.Line.Enable", "Child Text"=["False", "Read/Write", "Bool", "", "", "", "[0].RW.Bool.port1/line5.NI.Line.Enable", "DIO line output enable", "DIO output enable for one line. When a line is enabled, the input and output buffers for the front I/O connector and the rear I/O connector of the line are configured based on the NI.Line.Direction property. When a line is not enabled, the buffers for both the front I/O connector and the rear I/O connector are configured as inputs. Changes to this property take effect after running the NI.ChannelConfigurationUpdate command."], "Child Tag"="Physical Channel/port1/line5/Properties/NI.Line.Enable", "Item Indent"=3, "Child Only?"=FALSE, "Glyph Index"=9}, {"Left Cell String"="SLSC-12001-030EE1BC-Mod8/port1/line6", "Child Text"=[], "Child Tag"="Physical Channel/port1/line6", "Item Indent"=1, "Child Only?"=FALSE, "Glyph Index"=31}, {"Left Cell String"="Commands", "Child Text"=[], "Child Tag"="Physical Channel/port1/line6/Commands", "Item Indent"=2, "Child Only?"=FALSE, "Glyph Index"=35}, {"Left Cell String"="Properties", "Child Text"=[], "Child Tag"="Physical Channel/port1/line6/Properties", "Item Indent"=2, "Child Only?"=FALSE, "Glyph Index"=36}, {"Left Cell String"="NI.Line.Index", "Child Text"=["E", "Read Only", "U32", "", "", "", "[14].R.U32.port1/line6.NI.Line.Index", "Overall index of this DIO line in the module", "This is the index of this DIO line for the aggregate module properties: NI.FrontInputBufferState, NI.RearInputBufferState, and NI.TestModeValue."], "Child Tag"="Physical Channel/port1/line6/Properties/NI.Line.Index", "Item Indent"=3, "Child Only?"=FALSE, "Glyph Index"=8}, {"Left Cell String"="NI.Line.Direction", "Child Text"=["[0]Input", "Read/Write", "I32", "Enum", "NI.Line.Direction", "[0]Input;[1]Output_Source;[2]Output_Sink;[3]Output_PushPull;", "[0].RW.I32.port1/line6.NI.Line.Direction", "DIO line direction", "Line signal flow direction through the module, relative to the front I/O connector. This property is only used when the NI.ChannelEnable for this line is set to true. Changes to this property take effect after running the NI.ChannelConfigurationUpdate command."], "Child Tag"="Physical Channel/port1/line6/Properties/NI.Line.Direction", "Item Indent"=3, "Child Only?"=FALSE, "Glyph Index"=9}, {"Left Cell String"="NI.Line.Enable", "Child Text"=["False", "Read/Write", "Bool", "", "", "", "[0].RW.Bool.port1/line6.NI.Line.Enable", "DIO line output enable", "DIO output enable for one line. When a line is enabled, the input and output buffers for the front I/O connector and the rear I/O connector of the line are configured based on the NI.Line.Direction property. When a line is not enabled, the buffers for both the front I/O connector and the rear I/O connector are configured as inputs. Changes to this property take effect after running the NI.ChannelConfigurationUpdate command."], "Child Tag"="Physical Channel/port1/line6/Properties/NI.Line.Enable", "Item Indent"=3, "Child Only?"=FALSE, "Glyph Index"=9}, {"Left Cell String"="SLSC-12001-030EE1BC-Mod8/port1/line7", "Child Text"=[], "Child Tag"="Physical Channel/port1/line7", "Item Indent"=1, "Child Only?"=FALSE, "Glyph Index"=31}, {"Left Cell String"="Commands", "Child Text"=[], "Child Tag"="Physical Channel/port1/line7/Commands", "Item Indent"=2, "Child Only?"=FALSE, "Glyph Index"=35}, {"Left Cell String"="Properties", "Child Text"=[], "Child Tag"="Physical Channel/port1/line7/Properties", "Item Indent"=2, "Child Only?"=FALSE, "Glyph Index"=36}, {"Left Cell String"="NI.Line.Index", "Child Text"=["F", "Read Only", "U32", "", "", "", "[15].R.U32.port1/line7.NI.Line.Index", "Overall index of this DIO line in the module", "This is the index of this DIO line for the aggregate module properties: NI.FrontInputBufferState, NI.RearInputBufferState, and NI.TestModeValue."], "Child Tag"="Physical Channel/port1/line7/Properties/NI.Line.Index", "Item Indent"=3, "Child Only?"=FALSE, "Glyph Index"=8}, {"Left Cell String"="NI.Line.Direction", "Child Text"=["[0]Input", "Read/Write", "I32", "Enum", "NI.Line.Direction", "[0]Input;[1]Output_Source;[2]Output_Sink;[3]Output_PushPull;", "[0].RW.I32.port1/line7.NI.Line.Direction", "DIO line direction", "Line signal flow direction through the module, relative to the front I/O connector. This property is only used when the NI.ChannelEnable for this line is set to true. Changes to this property take effect after running the NI.ChannelConfigurationUpdate command."], "Child Tag"="Physical Channel/port1/line7/Properties/NI.Line.Direction", "Item Indent"=3, "Child Only?"=FALSE, "Glyph Index"=9}, {"Left Cell String"="NI.Line.Enable", "Child Text"=["False", "Read/Write", "Bool", "", "", "", "[0].RW.Bool.port1/line7.NI.Line.Enable", "DIO line output enable", "DIO output enable for one line. When a line is enabled, the input and output buffers for the front I/O connector and the rear I/O connector of the line are configured based on the NI.Line.Direction property. When a line is not enabled, the buffers for both the front I/O connector and the rear I/O connector are configured as inputs. Changes to this property take effect after running the NI.ChannelConfigurationUpdate command."], "Child Tag"="Physical Channel/port1/line7/Properties/NI.Line.Enable", "Item Indent"=3, "Child Only?"=FALSE, "Glyph Index"=9}, {"Left Cell String"="SLSC-12001-030EE1BC-Mod8/port2/line0", "Child Text"=[], "Child Tag"="Physical Channel/port2/line0", "Item Indent"=1, "Child Only?"=FALSE, "Glyph Index"=31}, {"Left Cell String"="Commands", "Child Text"=[], "Child Tag"="Physical Channel/port2/line0/Commands", "Item Indent"=2, "Child Only?"=FALSE, "Glyph Index"=35}, {"Left Cell String"="Properties", "Child Text"=[], "Child Tag"="Physical Channel/port2/line0/Properties", "Item Indent"=2, "Child Only?"=FALSE, "Glyph Index"=36}, {"Left Cell String"="NI.Line.Index", "Child Text"=["10", "Read Only", "U32", "", "", "", "[16].R.U32.port2/line0.NI.Line.Index", "Overall index of this DIO line in the module", "This is the index of this DIO line for the aggregate module properties: NI.FrontInputBufferState, NI.RearInputBufferState, and NI.TestModeValue."], "Child Tag"="Physical Channel/port2/line0/Properties/NI.Line.Index", "Item Indent"=3, "Child Only?"=FALSE, "Glyph Index"=8}, {"Left Cell String"="NI.Line.Direction", "Child Text"=["[0]Input", "Read/Write", "I32", "Enum", "NI.Line.Direction", "[0]Input;[1]Output_Source;[2]Output_Sink;[3]Output_PushPull;", "[0].RW.I32.port2/line0.NI.Line.Direction", "DIO line direction", "Line signal flow direction through the module, relative to the front I/O connector. This property is only used when the NI.ChannelEnable for this line is set to true. Changes to this property take effect after running the NI.ChannelConfigurationUpdate command."], "Child Tag"="Physical Channel/port2/line0/Properties/NI.Line.Direction", "Item Indent"=3, "Child Only?"=FALSE, "Glyph Index"=9}, {"Left Cell String"="NI.Line.Enable", "Child Text"=["False", "Read/Write", "Bool", "", "", "", "[0].RW.Bool.port2/line0.NI.Line.Enable", "DIO line output enable", "DIO output enable for one line. When a line is enabled, the input and output buffers for the front I/O connector and the rear I/O connector of the line are configured based on the NI.Line.Direction property. When a line is not enabled, the buffers for both the front I/O connector and the rear I/O connector are configured as inputs. Changes to this property take effect after running the NI.ChannelConfigurationUpdate command."], "Child Tag"="Physical Channel/port2/line0/Properties/NI.Line.Enable", "Item Indent"=3, "Child Only?"=FALSE, "Glyph Index"=9}, {"Left Cell String"="SLSC-12001-030EE1BC-Mod8/port2/line1", "Child Text"=[], "Child Tag"="Physical Channel/port2/line1", "Item Indent"=1, "Child Only?"=FALSE, "Glyph Index"=31}, {"Left Cell String"="Commands", "Child Text"=[], "Child Tag"="Physical Channel/port2/line1/Commands", "Item Indent"=2, "Child Only?"=FALSE, "Glyph Index"=35}, {"Left Cell String"="Properties", "Child Text"=[], "Child Tag"="Physical Channel/port2/line1/Properties", "Item Indent"=2, "Child Only?"=FALSE, "Glyph Index"=36}, {"Left Cell String"="NI.Line.Index", "Child Text"=["11", "Read Only", "U32", "", "", "", "[17].R.U32.port2/line1.NI.Line.Index", "Overall index of this DIO line in the module", "This is the index of this DIO line for the aggregate module properties: NI.FrontInputBufferState, NI.RearInputBufferState, and NI.TestModeValue."], "Child Tag"="Physical Channel/port2/line1/Properties/NI.Line.Index", "Item Indent"=3, "Child Only?"=FALSE, "Glyph Index"=8}, {"Left Cell String"="NI.Line.Direction", "Child Text"=["[0]Input", "Read/Write", "I32", "Enum", "NI.Line.Direction", "[0]Input;[1]Output_Source;[2]Output_Sink;[3]Output_PushPull;", "[0].RW.I32.port2/line1.NI.Line.Direction", "DIO line direction", "Line signal flow direction through the module, relative to the front I/O connector. This property is only used when the NI.ChannelEnable for this line is set to true. Changes to this property take effect after running the NI.ChannelConfigurationUpdate command."], "Child Tag"="Physical Channel/port2/line1/Properties/NI.Line.Direction", "Item Indent"=3, "Child Only?"=FALSE, "Glyph Index"=9}, {"Left Cell String"="NI.Line.Enable", "Child Text"=["False", "Read/Write", "Bool", "", "", "", "[0].RW.Bool.port2/line1.NI.Line.Enable", "DIO line output enable", "DIO output enable for one line. When a line is enabled, the input and output buffers for the front I/O connector and the rear I/O connector of the line are configured based on the NI.Line.Direction property. When a line is not enabled, the buffers for both the front I/O connector and the rear I/O connector are configured as inputs. Changes to this property take effect after running the NI.ChannelConfigurationUpdate command."], "Child Tag"="Physical Channel/port2/line1/Properties/NI.Line.Enable", "Item Indent"=3, "Child Only?"=FALSE, "Glyph Index"=9}, {"Left Cell String"="SLSC-12001-030EE1BC-Mod8/port2/line2", "Child Text"=[], "Child Tag"="Physical Channel/port2/line2", "Item Indent"=1, "Child Only?"=FALSE, "Glyph Index"=31}, {"Left Cell String"="Commands", "Child Text"=[], "Child Tag"="Physical Channel/port2/line2/Commands", "Item Indent"=2, "Child Only?"=FALSE, "Glyph Index"=35}, {"Left Cell String"="Properties", "Child Text"=[], "Child Tag"="Physical Channel/port2/line2/Properties", "Item Indent"=2, "Child Only?"=FALSE, "Glyph Index"=36}, {"Left Cell String"="NI.Line.Index", "Child Text"=["12", "Read Only", "U32", "", "", "", "[18].R.U32.port2/line2.NI.Line.Index", "Overall index of this DIO line in the module", "This is the index of this DIO line for the aggregate module properties: NI.FrontInputBufferState, NI.RearInputBufferState, and NI.TestModeValue."], "Child Tag"="Physical Channel/port2/line2/Properties/NI.Line.Index", "Item Indent"=3, "Child Only?"=FALSE, "Glyph Index"=8}, {"Left Cell String"="NI.Line.Direction", "Child Text"=["[0]Input", "Read/Write", "I32", "Enum", "NI.Line.Direction", "[0]Input;[1]Output_Source;[2]Output_Sink;[3]Output_PushPull;", "[0].RW.I32.port2/line2.NI.Line.Direction", "DIO line direction", "Line signal flow direction through the module, relative to the front I/O connector. This property is only used when the NI.ChannelEnable for this line is set to true. Changes to this property take effect after running the NI.ChannelConfigurationUpdate command."], "Child Tag"="Physical Channel/port2/line2/Properties/NI.Line.Direction", "Item Indent"=3, "Child Only?"=FALSE, "Glyph Index"=9}, {"Left Cell String"="NI.Line.Enable", "Child Text"=["False", "Read/Write", "Bool", "", "", "", "[0].RW.Bool.port2/line2.NI.Line.Enable", "DIO line output enable", "DIO output enable for one line. When a line is enabled, the input and output buffers for the front I/O connector and the rear I/O connector of the line are configured based on the NI.Line.Direction property. When a line is not enabled, the buffers for both the front I/O connector and the rear I/O connector are configured as inputs. Changes to this property take effect after running the NI.ChannelConfigurationUpdate command."], "Child Tag"="Physical Channel/port2/line2/Properties/NI.Line.Enable", "Item Indent"=3, "Child Only?"=FALSE, "Glyph Index"=9}, {"Left Cell String"="SLSC-12001-030EE1BC-Mod8/port2/line3", "Child Text"=[], "Child Tag"="Physical Channel/port2/line3", "Item Indent"=1, "Child Only?"=FALSE, "Glyph Index"=31}, {"Left Cell String"="Commands", "Child Text"=[], "Child Tag"="Physical Channel/port2/line3/Commands", "Item Indent"=2, "Child Only?"=FALSE, "Glyph Index"=35}, {"Left Cell String"="Properties", "Child Text"=[], "Child Tag"="Physical Channel/port2/line3/Properties", "Item Indent"=2, "Child Only?"=FALSE, "Glyph Index"=36}, {"Left Cell String"="NI.Line.Index", "Child Text"=["13", "Read Only", "U32", "", "", "", "[19].R.U32.port2/line3.NI.Line.Index", "Overall index of this DIO line in the module", "This is the index of this DIO line for the aggregate module properties: NI.FrontInputBufferState, NI.RearInputBufferState, and NI.TestModeValue."], "Child Tag"="Physical Channel/port2/line3/Properties/NI.Line.Index", "Item Indent"=3, "Child Only?"=FALSE, "Glyph Index"=8}, {"Left Cell String"="NI.Line.Direction", "Child Text"=["[0]Input", "Read/Write", "I32", "Enum", "NI.Line.Direction", "[0]Input;[1]Output_Source;[2]Output_Sink;[3]Output_PushPull;", "[0].RW.I32.port2/line3.NI.Line.Direction", "DIO line direction", "Line signal flow direction through the module, relative to the front I/O connector. This property is only used when the NI.ChannelEnable for this line is set to true. Changes to this property take effect after running the NI.ChannelConfigurationUpdate command."], "Child Tag"="Physical Channel/port2/line3/Properties/NI.Line.Direction", "Item Indent"=3, "Child Only?"=FALSE, "Glyph Index"=9}, {"Left Cell String"="NI.Line.Enable", "Child Text"=["False", "Read/Write", "Bool", "", "", "", "[0].RW.Bool.port2/line3.NI.Line.Enable", "DIO line output enable", "DIO output enable for one line. When a line is enabled, the input and output buffers for the front I/O connector and the rear I/O connector of the line are configured based on the NI.Line.Direction property. When a line is not enabled, the buffers for both the front I/O connector and the rear I/O connector are configured as inputs. Changes to this property take effect after running the NI.ChannelConfigurationUpdate command."], "Child Tag"="Physical Channel/port2/line3/Properties/NI.Line.Enable", "Item Indent"=3, "Child Only?"=FALSE, "Glyph Index"=9}, {"Left Cell String"="SLSC-12001-030EE1BC-Mod8/port2/line4", "Child Text"=[], "Child Tag"="Physical Channel/port2/line4", "Item Indent"=1, "Child Only?"=FALSE, "Glyph Index"=31}, {"Left Cell String"="Commands", "Child Text"=[], "Child Tag"="Physical Channel/port2/line4/Commands", "Item Indent"=2, "Child Only?"=FALSE, "Glyph Index"=35}, {"Left Cell String"="Properties", "Child Text"=[], "Child Tag"="Physical Channel/port2/line4/Properties", "Item Indent"=2, "Child Only?"=FALSE, "Glyph Index"=36}, {"Left Cell String"="NI.Line.Index", "Child Text"=["14", "Read Only", "U32", "", "", "", "[20].R.U32.port2/line4.NI.Line.Index", "Overall index of this DIO line in the module", "This is the index of this DIO line for the aggregate module properties: NI.FrontInputBufferState, NI.RearInputBufferState, and NI.TestModeValue."], "Child Tag"="Physical Channel/port2/line4/Properties/NI.Line.Index", "Item Indent"=3, "Child Only?"=FALSE, "Glyph Index"=8}, {"Left Cell String"="NI.Line.Direction", "Child Text"=["[0]Input", "Read/Write", "I32", "Enum", "NI.Line.Direction", "[0]Input;[1]Output_Source;[2]Output_Sink;[3]Output_PushPull;", "[0].RW.I32.port2/line4.NI.Line.Direction", "DIO line direction", "Line signal flow direction through the module, relative to the front I/O connector. This property is only used when the NI.ChannelEnable for this line is set to true. Changes to this property take effect after running the NI.ChannelConfigurationUpdate command."], "Child Tag"="Physical Channel/port2/line4/Properties/NI.Line.Direction", "Item Indent"=3, "Child Only?"=FALSE, "Glyph Index"=9}, {"Left Cell String"="NI.Line.Enable", "Child Text"=["False", "Read/Write", "Bool", "", "", "", "[0].RW.Bool.port2/line4.NI.Line.Enable", "DIO line output enable", "DIO output enable for one line. When a line is enabled, the input and output buffers for the front I/O connector and the rear I/O connector of the line are configured based on the NI.Line.Direction property. When a line is not enabled, the buffers for both the front I/O connector and the rear I/O connector are configured as inputs. Changes to this property take effect after running the NI.ChannelConfigurationUpdate command."], "Child Tag"="Physical Channel/port2/line4/Properties/NI.Line.Enable", "Item Indent"=3, "Child Only?"=FALSE, "Glyph Index"=9}, {"Left Cell String"="SLSC-12001-030EE1BC-Mod8/port2/line5", "Child Text"=[], "Child Tag"="Physical Channel/port2/line5", "Item Indent"=1, "Child Only?"=FALSE, "Glyph Index"=31}, {"Left Cell String"="Commands", "Child Text"=[], "Child Tag"="Physical Channel/port2/line5/Commands", "Item Indent"=2, "Child Only?"=FALSE, "Glyph Index"=35}, {"Left Cell String"="Properties", "Child Text"=[], "Child Tag"="Physical Channel/port2/line5/Properties", "Item Indent"=2, "Child Only?"=FALSE, "Glyph Index"=36}, {"Left Cell String"="NI.Line.Index", "Child Text"=["15", "Read Only", "U32", "", "", "", "[21].R.U32.port2/line5.NI.Line.Index", "Overall index of this DIO line in the module", "This is the index of this DIO line for the aggregate module properties: NI.FrontInputBufferState, NI.RearInputBufferState, and NI.TestModeValue."], "Child Tag"="Physical Channel/port2/line5/Properties/NI.Line.Index", "Item Indent"=3, "Child Only?"=FALSE, "Glyph Index"=8}, {"Left Cell String"="NI.Line.Direction", "Child Text"=["[0]Input", "Read/Write", "I32", "Enum", "NI.Line.Direction", "[0]Input;[1]Output_Source;[2]Output_Sink;[3]Output_PushPull;", "[0].RW.I32.port2/line5.NI.Line.Direction", "DIO line direction", "Line signal flow direction through the module, relative to the front I/O connector. This property is only used when the NI.ChannelEnable for this line is set to true. Changes to this property take effect after running the NI.ChannelConfigurationUpdate command."], "Child Tag"="Physical Channel/port2/line5/Properties/NI.Line.Direction", "Item Indent"=3, "Child Only?"=FALSE, "Glyph Index"=9}, {"Left Cell String"="NI.Line.Enable", "Child Text"=["False", "Read/Write", "Bool", "", "", "", "[0].RW.Bool.port2/line5.NI.Line.Enable", "DIO line output enable", "DIO output enable for one line. When a line is enabled, the input and output buffers for the front I/O connector and the rear I/O connector of the line are configured based on the NI.Line.Direction property. When a line is not enabled, the buffers for both the front I/O connector and the rear I/O connector are configured as inputs. Changes to this property take effect after running the NI.ChannelConfigurationUpdate command."], "Child Tag"="Physical Channel/port2/line5/Properties/NI.Line.Enable", "Item Indent"=3, "Child Only?"=FALSE, "Glyph Index"=9}, {"Left Cell String"="SLSC-12001-030EE1BC-Mod8/port2/line6", "Child Text"=[], "Child Tag"="Physical Channel/port2/line6", "Item Indent"=1, "Child Only?"=FALSE, "Glyph Index"=31}, {"Left Cell String"="Commands", "Child Text"=[], "Child Tag"="Physical Channel/port2/line6/Commands", "Item Indent"=2, "Child Only?"=FALSE, "Glyph Index"=35}, {"Left Cell String"="Properties", "Child Text"=[], "Child Tag"="Physical Channel/port2/line6/Properties", "Item Indent"=2, "Child Only?"=FALSE, "Glyph Index"=36}, {"Left Cell String"="NI.Line.Index", "Child Text"=["16", "Read Only", "U32", "", "", "", "[22].R.U32.port2/line6.NI.Line.Index", "Overall index of this DIO line in the module", "This is the index of this DIO line for the aggregate module properties: NI.FrontInputBufferState, NI.RearInputBufferState, and NI.TestModeValue."], "Child Tag"="Physical Channel/port2/line6/Properties/NI.Line.Index", "Item Indent"=3, "Child Only?"=FALSE, "Glyph Index"=8}, {"Left Cell String"="NI.Line.Direction", "Child Text"=["[0]Input", "Read/Write", "I32", "Enum", "NI.Line.Direction", "[0]Input;[1]Output_Source;[2]Output_Sink;[3]Output_PushPull;", "[0].RW.I32.port2/line6.NI.Line.Direction", "DIO line direction", "Line signal flow direction through the module, relative to the front I/O connector. This property is only used when the NI.ChannelEnable for this line is set to true. Changes to this property take effect after running the NI.ChannelConfigurationUpdate command."], "Child Tag"="Physical Channel/port2/line6/Properties/NI.Line.Direction", "Item Indent"=3, "Child Only?"=FALSE, "Glyph Index"=9}, {"Left Cell String"="NI.Line.Enable", "Child Text"=["False", "Read/Write", "Bool", "", "", "", "[0].RW.Bool.port2/line6.NI.Line.Enable", "DIO line output enable", "DIO output enable for one line. When a line is enabled, the input and output buffers for the front I/O connector and the rear I/O connector of the line are configured based on the NI.Line.Direction property. When a line is not enabled, the buffers for both the front I/O connector and the rear I/O connector are configured as inputs. Changes to this property take effect after running the NI.ChannelConfigurationUpdate command."], "Child Tag"="Physical Channel/port2/line6/Properties/NI.Line.Enable", "Item Indent"=3, "Child Only?"=FALSE, "Glyph Index"=9}, {"Left Cell String"="SLSC-12001-030EE1BC-Mod8/port2/line7", "Child Text"=[], "Child Tag"="Physical Channel/port2/line7", "Item Indent"=1, "Child Only?"=FALSE, "Glyph Index"=31}, {"Left Cell String"="Commands", "Child Text"=[], "Child Tag"="Physical Channel/port2/line7/Commands", "Item Indent"=2, "Child Only?"=FALSE, "Glyph Index"=35}, {"Left Cell String"="Properties", "Child Text"=[], "Child Tag"="Physical Channel/port2/line7/Properties", "Item Indent"=2, "Child Only?"=FALSE, "Glyph Index"=36}, {"Left Cell String"="NI.Line.Index", "Child Text"=["17", "Read Only", "U32", "", "", "", "[23].R.U32.port2/line7.NI.Line.Index", "Overall index of this DIO line in the module", "This is the index of this DIO line for the aggregate module properties: NI.FrontInputBufferState, NI.RearInputBufferState, and NI.TestModeValue."], "Child Tag"="Physical Channel/port2/line7/Properties/NI.Line.Index", "Item Indent"=3, "Child Only?"=FALSE, "Glyph Index"=8}, {"Left Cell String"="NI.Line.Direction", "Child Text"=["[0]Input", "Read/Write", "I32", "Enum", "NI.Line.Direction", "[0]Input;[1]Output_Source;[2]Output_Sink;[3]Output_PushPull;", "[0].RW.I32.port2/line7.NI.Line.Direction", "DIO line direction", "Line signal flow direction through the module, relative to the front I/O connector. This property is only used when the NI.ChannelEnable for this line is set to true. Changes to this property take effect after running the NI.ChannelConfigurationUpdate command."], "Child Tag"="Physical Channel/port2/line7/Properties/NI.Line.Direction", "Item Indent"=3, "Child Only?"=FALSE, "Glyph Index"=9}, {"Left Cell String"="NI.Line.Enable", "Child Text"=["False", "Read/Write", "Bool", "", "", "", "[0].RW.Bool.port2/line7.NI.Line.Enable", "DIO line output enable", "DIO output enable for one line. When a line is enabled, the input and output buffers for the front I/O connector and the rear I/O connector of the line are configured based on the NI.Line.Direction property. When a line is not enabled, the buffers for both the front I/O connector and the rear I/O connector are configured as inputs. Changes to this property take effect after running the NI.ChannelConfigurationUpdate command."], "Child Tag"="Physical Channel/port2/line7/Properties/NI.Line.Enable", "Item Indent"=3, "Child Only?"=FALSE, "Glyph Index"=9}, {"Left Cell String"="SLSC-12001-030EE1BC-Mod8/port3/line0", "Child Text"=[], "Child Tag"="Physical Channel/port3/line0", "Item Indent"=1, "Child Only?"=FALSE, "Glyph Index"=31}, {"Left Cell String"="Commands", "Child Text"=[], "Child Tag"="Physical Channel/port3/line0/Commands", "Item Indent"=2, "Child Only?"=FALSE, "Glyph Index"=35}, {"Left Cell String"="Properties", "Child Text"=[], "Child Tag"="Physical Channel/port3/line0/Properties", "Item Indent"=2, "Child Only?"=FALSE, "Glyph Index"=36}, {"Left Cell String"="NI.Line.Index", "Child Text"=["18", "Read Only", "U32", "", "", "", "[24].R.U32.port3/line0.NI.Line.Index", "Overall index of this DIO line in the module", "This is the index of this DIO line for the aggregate module properties: NI.FrontInputBufferState, NI.RearInputBufferState, and NI.TestModeValue."], "Child Tag"="Physical Channel/port3/line0/Properties/NI.Line.Index", "Item Indent"=3, "Child Only?"=FALSE, "Glyph Index"=8}, {"Left Cell String"="NI.Line.Direction", "Child Text"=["[0]Input", "Read/Write", "I32", "Enum", "NI.Line.Direction", "[0]Input;[1]Output_Source;[2]Output_Sink;[3]Output_PushPull;", "[0].RW.I32.port3/line0.NI.Line.Direction", "DIO line direction", "Line signal flow direction through the module, relative to the front I/O connector. This property is only used when the NI.ChannelEnable for this line is set to true. Changes to this property take effect after running the NI.ChannelConfigurationUpdate command."], "Child Tag"="Physical Channel/port3/line0/Properties/NI.Line.Direction", "Item Indent"=3, "Child Only?"=FALSE, "Glyph Index"=9}, {"Left Cell String"="NI.Line.Enable", "Child Text"=["False", "Read/Write", "Bool", "", "", "", "[0].RW.Bool.port3/line0.NI.Line.Enable", "DIO line output enable", "DIO output enable for one line. When a line is enabled, the input and output buffers for the front I/O connector and the rear I/O connector of the line are configured based on the NI.Line.Direction property. When a line is not enabled, the buffers for both the front I/O connector and the rear I/O connector are configured as inputs. Changes to this property take effect after running the NI.ChannelConfigurationUpdate command."], "Child Tag"="Physical Channel/port3/line0/Properties/NI.Line.Enable", "Item Indent"=3, "Child Only?"=FALSE, "Glyph Index"=9}, {"Left Cell String"="SLSC-12001-030EE1BC-Mod8/port3/line1", "Child Text"=[], "Child Tag"="Physical Channel/port3/line1", "Item Indent"=1, "Child Only?"=FALSE, "Glyph Index"=31}, {"Left Cell String"="Commands", "Child Text"=[], "Child Tag"="Physical Channel/port3/line1/Commands", "Item Indent"=2, "Child Only?"=FALSE, "Glyph Index"=35}, {"Left Cell String"="Properties", "Child Text"=[], "Child Tag"="Physical Channel/port3/line1/Properties", "Item Indent"=2, "Child Only?"=FALSE, "Glyph Index"=36}, {"Left Cell String"="NI.Line.Index", "Child Text"=["19", "Read Only", "U32", "", "", "", "[25].R.U32.port3/line1.NI.Line.Index", "Overall index of this DIO line in the module", "This is the index of this DIO line for the aggregate module properties: NI.FrontInputBufferState, NI.RearInputBufferState, and NI.TestModeValue."], "Child Tag"="Physical Channel/port3/line1/Properties/NI.Line.Index", "Item Indent"=3, "Child Only?"=FALSE, "Glyph Index"=8}, {"Left Cell String"="NI.Line.Direction", "Child Text"=["[0]Input", "Read/Write", "I32", "Enum", "NI.Line.Direction", "[0]Input;[1]Output_Source;[2]Output_Sink;[3]Output_PushPull;", "[0].RW.I32.port3/line1.NI.Line.Direction", "DIO line direction", "Line signal flow direction through the module, relative to the front I/O connector. This property is only used when the NI.ChannelEnable for this line is set to true. Changes to this property take effect after running the NI.ChannelConfigurationUpdate command."], "Child Tag"="Physical Channel/port3/line1/Properties/NI.Line.Direction", "Item Indent"=3, "Child Only?"=FALSE, "Glyph Index"=9}, {"Left Cell String"="NI.Line.Enable", "Child Text"=["False", "Read/Write", "Bool", "", "", "", "[0].RW.Bool.port3/line1.NI.Line.Enable", "DIO line output enable", "DIO output enable for one line. When a line is enabled, the input and output buffers for the front I/O connector and the rear I/O connector of the line are configured based on the NI.Line.Direction property. When a line is not enabled, the buffers for both the front I/O connector and the rear I/O connector are configured as inputs. Changes to this property take effect after running the NI.ChannelConfigurationUpdate command."], "Child Tag"="Physical Channel/port3/line1/Properties/NI.Line.Enable", "Item Indent"=3, "Child Only?"=FALSE, "Glyph Index"=9}, {"Left Cell String"="SLSC-12001-030EE1BC-Mod8/port3/line2", "Child Text"=[], "Child Tag"="Physical Channel/port3/line2", "Item Indent"=1, "Child Only?"=FALSE, "Glyph Index"=31}, {"Left Cell String"="Commands", "Child Text"=[], "Child Tag"="Physical Channel/port3/line2/Commands", "Item Indent"=2, "Child Only?"=FALSE, "Glyph Index"=35}, {"Left Cell String"="Properties", "Child Text"=[], "Child Tag"="Physical Channel/port3/line2/Properties", "Item Indent"=2, "Child Only?"=FALSE, "Glyph Index"=36}, {"Left Cell String"="NI.Line.Index", "Child Text"=["1A", "Read Only", "U32", "", "", "", "[26].R.U32.port3/line2.NI.Line.Index", "Overall index of this DIO line in the module", "This is the index of this DIO line for the aggregate module properties: NI.FrontInputBufferState, NI.RearInputBufferState, and NI.TestModeValue."], "Child Tag"="Physical Channel/port3/line2/Properties/NI.Line.Index", "Item Indent"=3, "Child Only?"=FALSE, "Glyph Index"=8}, {"Left Cell String"="NI.Line.Direction", "Child Text"=["[0]Input", "Read/Write", "I32", "Enum", "NI.Line.Direction", "[0]Input;[1]Output_Source;[2]Output_Sink;[3]Output_PushPull;", "[0].RW.I32.port3/line2.NI.Line.Direction", "DIO line direction", "Line signal flow direction through the module, relative to the front I/O connector. This property is only used when the NI.ChannelEnable for this line is set to true. Changes to this property take effect after running the NI.ChannelConfigurationUpdate command."], "Child Tag"="Physical Channel/port3/line2/Properties/NI.Line.Direction", "Item Indent"=3, "Child Only?"=FALSE, "Glyph Index"=9}, {"Left Cell String"="NI.Line.Enable", "Child Text"=["False", "Read/Write", "Bool", "", "", "", "[0].RW.Bool.port3/line2.NI.Line.Enable", "DIO line output enable", "DIO output enable for one line. When a line is enabled, the input and output buffers for the front I/O connector and the rear I/O connector of the line are configured based on the NI.Line.Direction property. When a line is not enabled, the buffers for both the front I/O connector and the rear I/O connector are configured as inputs. Changes to this property take effect after running the NI.ChannelConfigurationUpdate command."], "Child Tag"="Physical Channel/port3/line2/Properties/NI.Line.Enable", "Item Indent"=3, "Child Only?"=FALSE, "Glyph Index"=9}, {"Left Cell String"="SLSC-12001-030EE1BC-Mod8/port3/line3", "Child Text"=[], "Child Tag"="Physical Channel/port3/line3", "Item Indent"=1, "Child Only?"=FALSE, "Glyph Index"=31}, {"Left Cell String"="Commands", "Child Text"=[], "Child Tag"="Physical Channel/port3/line3/Commands", "Item Indent"=2, "Child Only?"=FALSE, "Glyph Index"=35}, {"Left Cell String"="Properties", "Child Text"=[], "Child Tag"="Physical Channel/port3/line3/Properties", "Item Indent"=2, "Child Only?"=FALSE, "Glyph Index"=36}, {"Left Cell String"="NI.Line.Index", "Child Text"=["1B", "Read Only", "U32", "", "", "", "[27].R.U32.port3/line3.NI.Line.Index", "Overall index of this DIO line in the module", "This is the index of this DIO line for the aggregate module properties: NI.FrontInputBufferState, NI.RearInputBufferState, and NI.TestModeValue."], "Child Tag"="Physical Channel/port3/line3/Properties/NI.Line.Index", "Item Indent"=3, "Child Only?"=FALSE, "Glyph Index"=8}, {"Left Cell String"="NI.Line.Direction", "Child Text"=["[0]Input", "Read/Write", "I32", "Enum", "NI.Line.Direction", "[0]Input;[1]Output_Source;[2]Output_Sink;[3]Output_PushPull;", "[0].RW.I32.port3/line3.NI.Line.Direction", "DIO line direction", "Line signal flow direction through the module, relative to the front I/O connector. This property is only used when the NI.ChannelEnable for this line is set to true. Changes to this property take effect after running the NI.ChannelConfigurationUpdate command."], "Child Tag"="Physical Channel/port3/line3/Properties/NI.Line.Direction", "Item Indent"=3, "Child Only?"=FALSE, "Glyph Index"=9}, {"Left Cell String"="NI.Line.Enable", "Child Text"=["False", "Read/Write", "Bool", "", "", "", "[0].RW.Bool.port3/line3.NI.Line.Enable", "DIO line output enable", "DIO output enable for one line. When a line is enabled, the input and output buffers for the front I/O connector and the rear I/O connector of the line are configured based on the NI.Line.Direction property. When a line is not enabled, the buffers for both the front I/O connector and the rear I/O connector are configured as inputs. Changes to this property take effect after running the NI.ChannelConfigurationUpdate command."], "Child Tag"="Physical Channel/port3/line3/Properties/NI.Line.Enable", "Item Indent"=3, "Child Only?"=FALSE, "Glyph Index"=9}, {"Left Cell String"="SLSC-12001-030EE1BC-Mod8/port3/line4", "Child Text"=[], "Child Tag"="Physical Channel/port3/line4", "Item Indent"=1, "Child Only?"=FALSE, "Glyph Index"=31}, {"Left Cell String"="Commands", "Child Text"=[], "Child Tag"="Physical Channel/port3/line4/Commands", "Item Indent"=2, "Child Only?"=FALSE, "Glyph Index"=35}, {"Left Cell String"="Properties", "Child Text"=[], "Child Tag"="Physical Channel/port3/line4/Properties", "Item Indent"=2, "Child Only?"=FALSE, "Glyph Index"=36}, {"Left Cell String"="NI.Line.Index", "Child Text"=["1C", "Read Only", "U32", "", "", "", "[28].R.U32.port3/line4.NI.Line.Index", "Overall index of this DIO line in the module", "This is the index of this DIO line for the aggregate module properties: NI.FrontInputBufferState, NI.RearInputBufferState, and NI.TestModeValue."], "Child Tag"="Physical Channel/port3/line4/Properties/NI.Line.Index", "Item Indent"=3, "Child Only?"=FALSE, "Glyph Index"=8}, {"Left Cell String"="NI.Line.Direction", "Child Text"=["[0]Input", "Read/Write", "I32", "Enum", "NI.Line.Direction", "[0]Input;[1]Output_Source;[2]Output_Sink;[3]Output_PushPull;", "[0].RW.I32.port3/line4.NI.Line.Direction", "DIO line direction", "Line signal flow direction through the module, relative to the front I/O connector. This property is only used when the NI.ChannelEnable for this line is set to true. Changes to this property take effect after running the NI.ChannelConfigurationUpdate command."], "Child Tag"="Physical Channel/port3/line4/Properties/NI.Line.Direction", "Item Indent"=3, "Child Only?"=FALSE, "Glyph Index"=9}, {"Left Cell String"="NI.Line.Enable", "Child Text"=["False", "Read/Write", "Bool", "", "", "", "[0].RW.Bool.port3/line4.NI.Line.Enable", "DIO line output enable", "DIO output enable for one line. When a line is enabled, the input and output buffers for the front I/O connector and the rear I/O connector of the line are configured based on the NI.Line.Direction property. When a line is not enabled, the buffers for both the front I/O connector and the rear I/O connector are configured as inputs. Changes to this property take effect after running the NI.ChannelConfigurationUpdate command."], "Child Tag"="Physical Channel/port3/line4/Properties/NI.Line.Enable", "Item Indent"=3, "Child Only?"=FALSE, "Glyph Index"=9}, {"Left Cell String"="SLSC-12001-030EE1BC-Mod8/port3/line5", "Child Text"=[], "Child Tag"="Physical Channel/port3/line5", "Item Indent"=1, "Child Only?"=FALSE, "Glyph Index"=31}, {"Left Cell String"="Commands", "Child Text"=[], "Child Tag"="Physical Channel/port3/line5/Commands", "Item Indent"=2, "Child Only?"=FALSE, "Glyph Index"=35}, {"Left Cell String"="Properties", "Child Text"=[], "Child Tag"="Physical Channel/port3/line5/Properties", "Item Indent"=2, "Child Only?"=FALSE, "Glyph Index"=36}, {"Left Cell String"="NI.Line.Index", "Child Text"=["1D", "Read Only", "U32", "", "", "", "[29].R.U32.port3/line5.NI.Line.Index", "Overall index of this DIO line in the module", "This is the index of this DIO line for the aggregate module properties: NI.FrontInputBufferState, NI.RearInputBufferState, and NI.TestModeValue."], "Child Tag"="Physical Channel/port3/line5/Properties/NI.Line.Index", "Item Indent"=3, "Child Only?"=FALSE, "Glyph Index"=8}, {"Left Cell String"="NI.Line.Direction", "Child Text"=["[0]Input", "Read/Write", "I32", "Enum", "NI.Line.Direction", "[0]Input;[1]Output_Source;[2]Output_Sink;[3]Output_PushPull;", "[0].RW.I32.port3/line5.NI.Line.Direction", "DIO line direction", "Line signal flow direction through the module, relative to the front I/O connector. This property is only used when the NI.ChannelEnable for this line is set to true. Changes to this property take effect after running the NI.ChannelConfigurationUpdate command."], "Child Tag"="Physical Channel/port3/line5/Properties/NI.Line.Direction", "Item Indent"=3, "Child Only?"=FALSE, "Glyph Index"=9}, {"Left Cell String"="NI.Line.Enable", "Child Text"=["False", "Read/Write", "Bool", "", "", "", "[0].RW.Bool.port3/line5.NI.Line.Enable", "DIO line output enable", "DIO output enable for one line. When a line is enabled, the input and output buffers for the front I/O connector and the rear I/O connector of the line are configured based on the NI.Line.Direction property. When a line is not enabled, the buffers for both the front I/O connector and the rear I/O connector are configured as inputs. Changes to this property take effect after running the NI.ChannelConfigurationUpdate command."], "Child Tag"="Physical Channel/port3/line5/Properties/NI.Line.Enable", "Item Indent"=3, "Child Only?"=FALSE, "Glyph Index"=9}, {"Left Cell String"="SLSC-12001-030EE1BC-Mod8/port3/line6", "Child Text"=[], "Child Tag"="Physical Channel/port3/line6", "Item Indent"=1, "Child Only?"=FALSE, "Glyph Index"=31}, {"Left Cell String"="Commands", "Child Text"=[], "Child Tag"="Physical Channel/port3/line6/Commands", "Item Indent"=2, "Child Only?"=FALSE, "Glyph Index"=35}, {"Left Cell String"="Properties", "Child Text"=[], "Child Tag"="Physical Channel/port3/line6/Properties", "Item Indent"=2, "Child Only?"=FALSE, "Glyph Index"=36}, {"Left Cell String"="NI.Line.Index", "Child Text"=["1E", "Read Only", "U32", "", "", "", "[30].R.U32.port3/line6.NI.Line.Index", "Overall index of this DIO line in the module", "This is the index of this DIO line for the aggregate module properties: NI.FrontInputBufferState, NI.RearInputBufferState, and NI.TestModeValue."], "Child Tag"="Physical Channel/port3/line6/Properties/NI.Line.Index", "Item Indent"=3, "Child Only?"=FALSE, "Glyph Index"=8}, {"Left Cell String"="NI.Line.Direction", "Child Text"=["[0]Input", "Read/Write", "I32", "Enum", "NI.Line.Direction", "[0]Input;[1]Output_Source;[2]Output_Sink;[3]Output_PushPull;", "[0].RW.I32.port3/line6.NI.Line.Direction", "DIO line direction", "Line signal flow direction through the module, relative to the front I/O connector. This property is only used when the NI.ChannelEnable for this line is set to true. Changes to this property take effect after running the NI.ChannelConfigurationUpdate command."], "Child Tag"="Physical Channel/port3/line6/Properties/NI.Line.Direction", "Item Indent"=3, "Child Only?"=FALSE, "Glyph Index"=9}, {"Left Cell String"="NI.Line.Enable", "Child Text"=["False", "Read/Write", "Bool", "", "", "", "[0].RW.Bool.port3/line6.NI.Line.Enable", "DIO line output enable", "DIO output enable for one line. When a line is enabled, the input and output buffers for the front I/O connector and the rear I/O connector of the line are configured based on the NI.Line.Direction property. When a line is not enabled, the buffers for both the front I/O connector and the rear I/O connector are configured as inputs. Changes to this property take effect after running the NI.ChannelConfigurationUpdate command."], "Child Tag"="Physical Channel/port3/line6/Properties/NI.Line.Enable", "Item Indent"=3, "Child Only?"=FALSE, "Glyph Index"=9}, {"Left Cell String"="SLSC-12001-030EE1BC-Mod8/port3/line7", "Child Text"=[], "Child Tag"="Physical Channel/port3/line7", "Item Indent"=1, "Child Only?"=FALSE, "Glyph Index"=31}, {"Left Cell String"="Commands", "Child Text"=[], "Child Tag"="Physical Channel/port3/line7/Commands", "Item Indent"=2, "Child Only?"=FALSE, "Glyph Index"=35}, {"Left Cell String"="Properties", "Child Text"=[], "Child Tag"="Physical Channel/port3/line7/Properties", "Item Indent"=2, "Child Only?"=FALSE, "Glyph Index"=36}, {"Left Cell String"="NI.Line.Index", "Child Text"=["1F", "Read Only", "U32", "", "", "", "[31].R.U32.port3/line7.NI.Line.Index", "Overall index of this DIO line in the module", "This is the index of this DIO line for the aggregate module properties: NI.FrontInputBufferState, NI.RearInputBufferState, and NI.TestModeValue."], "Child Tag"="Physical Channel/port3/line7/Properties/NI.Line.Index", "Item Indent"=3, "Child Only?"=FALSE, "Glyph Index"=8}, {"Left Cell String"="NI.Line.Direction", "Child Text"=["[0]Input", "Read/Write", "I32", "Enum", "NI.Line.Direction", "[0]Input;[1]Output_Source;[2]Output_Sink;[3]Output_PushPull;", "[0].RW.I32.port3/line7.NI.Line.Direction", "DIO line direction", "Line signal flow direction through the module, relative to the front I/O connector. This property is only used when the NI.ChannelEnable for this line is set to true. Changes to this property take effect after running the NI.ChannelConfigurationUpdate command."], "Child Tag"="Physical Channel/port3/line7/Properties/NI.Line.Direction", "Item Indent"=3, "Child Only?"=FALSE, "Glyph Index"=9}, {"Left Cell String"="NI.Line.Enable", "Child Text"=["False", "Read/Write", "Bool", "", "", "", "[0].RW.Bool.port3/line7.NI.Line.Enable", "DIO line output enable", "DIO output enable for one line. When a line is enabled, the input and output buffers for the front I/O connector and the rear I/O connector of the line are configured based on the NI.Line.Direction property. When a line is not enabled, the buffers for both the front I/O connector and the rear I/O connector are configured as inputs. Changes to this property take effect after running the NI.ChannelConfigurationUpdate command."], "Child Tag"="Physical Channel/port3/line7/Properties/NI.Line.Enable", "Item Indent"=3, "Child Only?"=FALSE, "Glyph Index"=9}], 7 "Channels to \"enable\"":string[](array[string]), 9 "Channel Values":dbl[](array[numeric]), 11 "error in (no error)":errorcluster, 13 "Enum Strings":cluster{"name":string, string}[](array[cluster])) -> (15 "error out":errorcluster)   [LabVIEW 2015, in "SLSC Tree Control.lvlib"]
doc: "Updates the tree control with the new information from the SLSC Output Tree. It also changes the icons according to to the state of the channel."
uses:
  SLSC Tree Control.lvlib
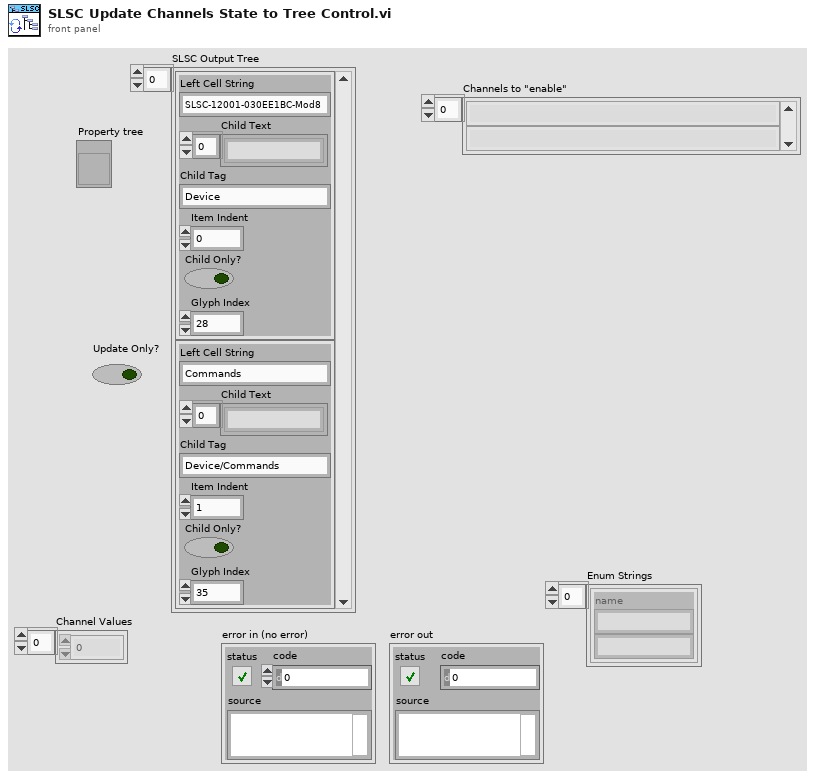
[diagram p1: front panel]
types:
  T1 = cluster{"Left Cell String":string, "Child Text":string[], "Child Tag":string, "Item Indent":i32, "Child Only?":bool, "Glyph Index":i32}[]
  T2 = cluster{"Left Cell String":string, "Child Text":string[], "Child Tag":string, "Item Indent":i32, "Child Only?":bool, "Glyph Index":i32}
  T3 = typedef "LVNodeAndColumnTypeDef.ctl" = cluster{"Node":string, "Column":i32}
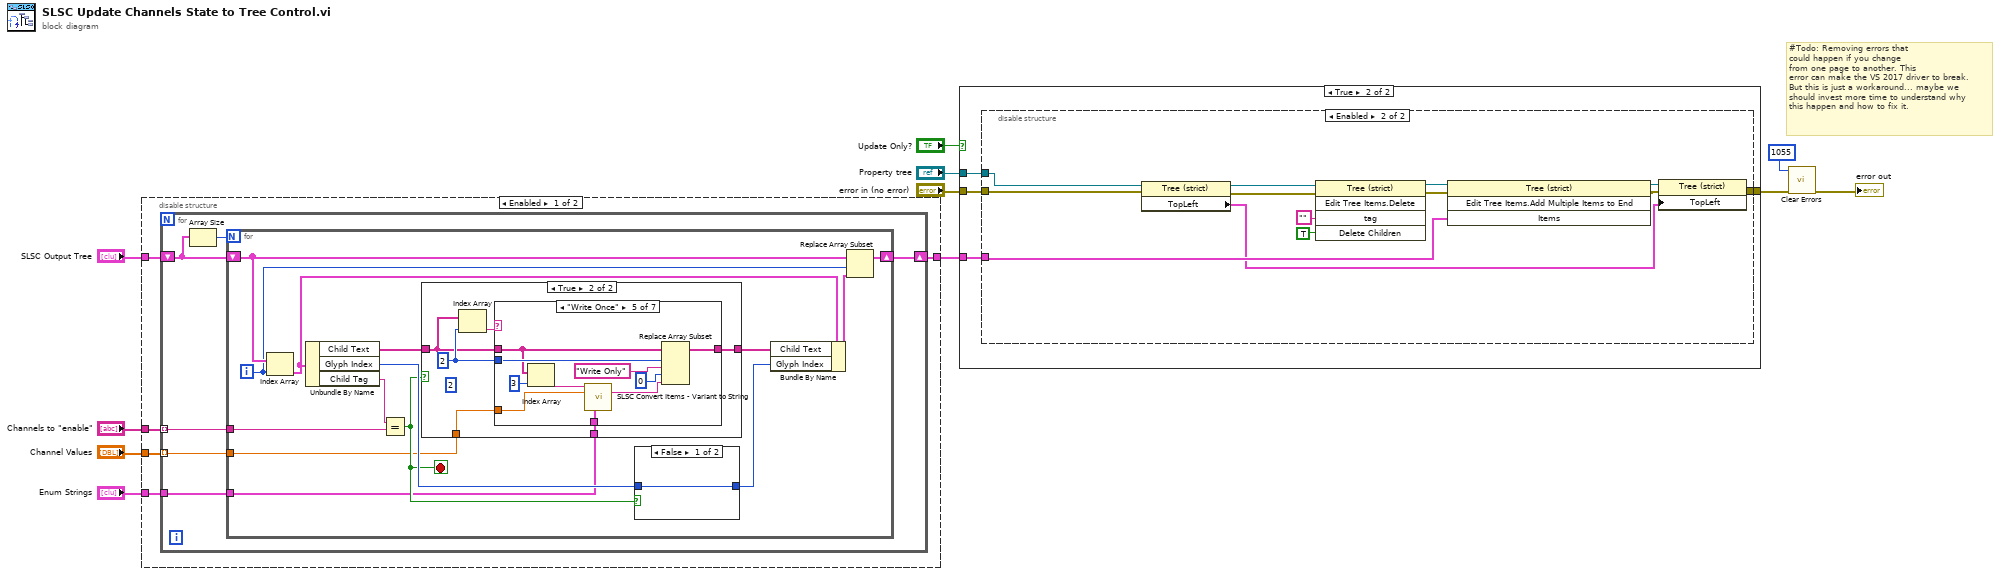
[diagram p0: block diagram]
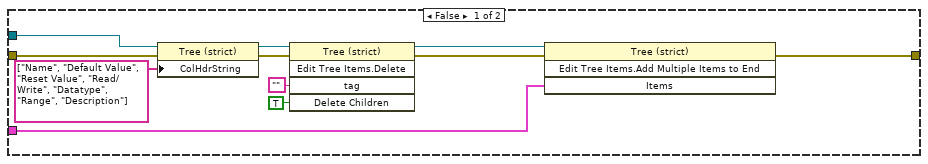
[diagram p2: hidden frame]
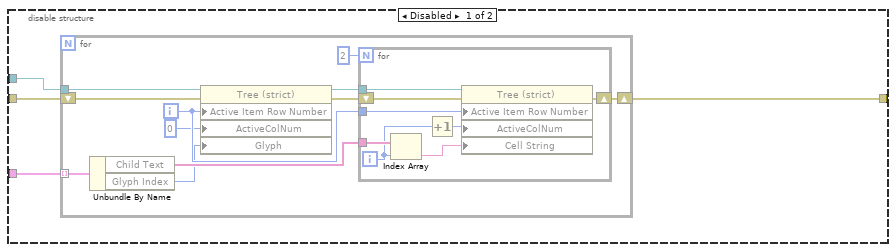
[diagram p3: hidden frame]
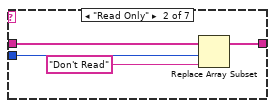
[diagram p6: hidden frame]
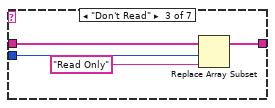
[diagram p7: hidden frame]
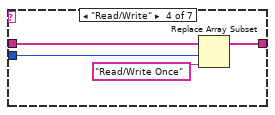
[diagram p8: hidden frame]
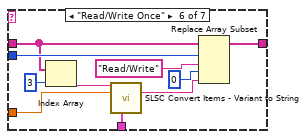
[diagram p9: hidden frame]
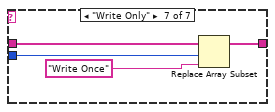
[diagram p10: hidden frame]
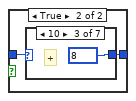
[diagram p11: hidden frame]
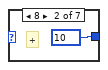
[diagram p13: hidden frame]
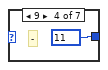
[diagram p14: hidden frame]
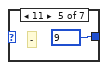
[diagram p15: hidden frame]
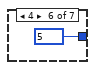
[diagram p16: hidden frame]
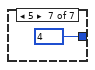
[diagram p17: hidden frame]
diagram:
  # "#Todo: Removing errors that\ncould happen if you change\nfrom one page to another. This \nerror can make the VS 2017 driver to break. \nBut this is just a workaround... maybe we \nshould invest more time to understand why\nthis happen and how to fix it."
  n1 = disable-structure shown="Enabled" {
    disable-tunnel: [w16 w91] -> w9
    disable-tunnel: "SLSC Output Tree" -> [w15 w91]
    disable-tunnel: "Channels to \"enable\"" -> [w14 _]
    disable-tunnel: "Channel Values" -> [w13 _]
    disable-tunnel: "Enum Strings" -> [w12 _]
    frame Enabled {
      n2 = for {
        tunnel: w14 -> [w19] mode=indexing
        shift-right: [w22] -> w16
        shift-left: w15 -> [w20]
        tunnel: w13 -> [w18] mode=indexing
        tunnel: w12 -> [w17]
        n3 = Array Size(array=w20) -> (size(s)=w21:i32)
        n4 = for {
          N: w21 -> [_]
          shift-right: [w35] -> w22
          shift-left: w20 -> [w36]
          tunnel: w19 -> [w31]
          tunnel: w18 -> [w24]
          tunnel: w17 -> [w23]
          i -> [w34]
          stop <- w27 stop-if-true
          n5 = Index Array(array=w36, index=w34) -> (element=w30:T2)
          n6 = Unbundle By Name(w30) -> ("Child Text"=w25:string[], "Glyph Index"=w28:i32, "Child Tag"=w32:string)
          n7 = Equal?(x=w32, y=w31) -> (x = y?=w27:bool)
          n8 = case shown="True" w27 {
            tunnel: [w37 w43] -> w26
            tunnel: w25 -> [w37 w41]
            tunnel: w24 -> [_ w39]
            tunnel: w23 -> [_ w38]
            frame False {
            }
            frame True {
              (unwired) 2 ("index")
              w42 = 2 ("index")
              n9 = Index Array(array=w41, index=w42) -> (element=w40:string)
              n10 = case shown="\"Write Once\"" w40 {
                tunnel: w41 -> [w44 w48 w52 w56 w63 w73 w80]
                tunnel: [w44 w47 w51 w55 w66 w76 w79] -> w43
                tunnel: w42 -> [_ w46 w50 w54 w65 w75 w78]
                tunnel: w39 -> [_ _ _ _ w60 w70 _]
                tunnel: w38 -> [_ _ _ _ w59 w69 _]
                frame Default {
                }
                frame "Read Only" {
                  n11 = Replace Array Subset(array=w48, new element="Don't Read" ("new element/subarray"), index=w46) -> (w47:string[])
                }
                frame "Don't Read" {
                  n12 = Replace Array Subset(array=w52, new element="Read Only" ("new element/subarray"), index=w50) -> (w51:string[])
                }
                frame "Read/Write" {
                  n13 = Replace Array Subset(array=w56, new element="Read/Write Once" ("new element/subarray"), index=w54) -> (w55:string[])
                }
                frame "Write Once" {
                  n14 = Index Array(array=w63, index=3) -> (element=w61:string)
                  n15 = call "SLSC Convert Items - Variant to String.vi"("Datatype"=w61, "value"=w60, "Enum string"=w59) -> ("string data value"=w58:string)  [unwired: 6 in, 6 out]
                  n16 = Replace Array Subset(array=w63, new element #1="Write Only" ("new element/subarray"), index #1=w65, new element #2=w58, index #2=0 ("index")) -> (w66:string[])
                }
                frame "Read/Write Once" {
                  n17 = Index Array(array=w73, index=3) -> (element=w71:string)
                  n18 = call "SLSC Convert Items - Variant to String.vi"("Datatype"=w71, "value"=w70, "Enum string"=w69) -> ("string data value"=w68:string)  [unwired: 6 in, 6 out]
                  n19 = Replace Array Subset(array=w73, new element #1="Read/Write" ("new element/subarray"), index #1=w75, new element #2=w68, index #2=0 ("index")) -> (w76:string[])
                }
                frame "Write Only" {
                  n20 = Replace Array Subset(array=w80, new element="Write Once" ("new element/subarray"), index=w78) -> (w79:string[])
                }
              }
            }
          }
          n21 = case shown="False" w27 {
            tunnel: [w81 w82] -> w29
            tunnel: w28 -> [w81 w83]
            frame False {
            }
            frame True {
              n22 = case shown="10" w83 {
                selector: w83 -> [w84 _ _ _ _ _ _]
                tunnel: [w84 10 8 11 9 5 4] -> w82
                frame Default {
                }
                frame 8 {
                  # "+"
                }
                frame 10 {
                  # "+"
                }
                frame 9 {
                  # "-"
                }
                frame 11 {
                  # "-"
                }
                frame 4 {
                }
                frame 5 {
                }
              }
            }
          }
          n23 = Bundle By Name(cluster=w30, "Child Text"=w26, "Glyph Index"=w29) -> (w33:T2)
          n24 = Replace Array Subset(array=w36, new element=w33, index=w34) -> (w35:T1)
        }
      }
    }
    frame Disabled {
    }
  }
  n25 = case shown="True" "Update Only?" {
    tunnel: "error in (no error)" -> [w97 w104]
    tunnel: [w94 w103] -> w3
    tunnel: "Property tree" -> [w96 w105]
    tunnel: w9 -> [w95 w106]
    frame False {
      n26 = property on="Property Node" class="Tree (strict)"(reference=w96, error in=w97, "ColHdrString"=string[] ["Name", "Default Value", "Reset Value", "Read/Write", "Datatype", "Range", "Description"]) -> (reference out=w98:refnum<vi>, error out=w99:errorcluster)
      n27 = invoke on="Invoke Node" class="Tree (strict)" method="Edit Tree Items.Delete"(reference=w98, error in=w99, "tag"="", "Delete Children"=TRUE ("Delete Children?")) -> (reference out=w93:refnum<vi>, error out=w92:errorcluster)  [unwired: 1 in, 3 out]
      n28 = invoke on="Invoke Node" class="Tree (strict)" method="Edit Tree Items.Add Multiple Items to End"(reference=w93, error in=w92, "Items"=w95) -> (error out=w94:errorcluster)  [unwired: 1 in, 3 out]
    }
    frame True {
      n29 = disable-structure shown="Enabled" {
        disable-tunnel: w106 -> [w110 w137]
        disable-tunnel: w105 -> [w109 w136]
        disable-tunnel: w104 -> [w108 w135]
        disable-tunnel: [w107 _] -> w103
        frame Disabled {
          n30 = for {
            tunnel: w110 -> [w120] mode=indexing
            tunnel: w109 -> [w118]
            shift-right: [w121] -> w107
            shift-left: w108 -> [w115]
            i -> [w114]
            n31 = Unbundle By Name(w120) -> ("Child Text"=w119:string[], "Glyph Index"=w112:i32)
            n32 = property class="Tree (strict)"(reference=w118, error in=w115, "Active Item Row Number"=w114, "ActiveColNum"=0 ("Active Cell:Active Column Number"), "Glyph"=w112) -> (reference out=w117:refnum<vi>, error out=w116:errorcluster)
            n33 = for {
              N: 2 -> [_]
              tunnel: w117 -> [w129]
              shift-right: [w127] -> w121
              shift-left: w116 -> [w128]
              tunnel: w114 -> [w125]
              tunnel: w119 -> [w126]
              i -> [w122]
              n34 = Index Array(array=w126, index=w122) -> (element=w123:string)
              n35 = Increment(x=w122) -> (x+1=w124:i32)
              n36 = property class="Tree (strict)"(reference=w129, error in=w128, "Active Item Row Number"=w125, "ActiveColNum"=w124, "Cell String"=w123) -> (error out=w127:errorcluster)  [unwired: 1 out]
            }
          }
        }
        frame Enabled {
          n37 = property on="Property Node" class="Tree (strict)"(reference=w136, error in=w135) -> (reference out=w132:refnum<vi>, error out=w131:errorcluster, "TopLeft"=w130:T3)
          n38 = invoke on="Invoke Node" class="Tree (strict)" method="Edit Tree Items.Delete"(reference=w132, error in=w131, "tag"="", "Delete Children"=TRUE ("Delete Children?")) -> (reference out=w133:refnum<vi>, error out=w134:errorcluster)  [unwired: 1 in, 3 out]
          n39 = invoke on="Invoke Node" class="Tree (strict)" method="Edit Tree Items.Add Multiple Items to End"(reference=w133, error in=w134, "Items"=w137) -> (reference out=w139:refnum<vi>, error out=w138:errorcluster)  [unwired: 1 in, 2 out]
          n40 = property on="Property Node" class="Tree (strict)"(reference=w139, error in=w138, "TopLeft"=w130) -> ()  [unwired: 2 out]
        }
      }
    }
  }
  n41 = call <vilib>:"Clear Errors.vi"("error in (no error)"=w3, "specific error code to clear (0: all)"=1055) -> ("error out"=→"error out":errorcluster)  [unwired: 4 in, 1 out]
